vi "test_GUI_with_seq.vi"(8 "Variables":T2=[{"Value"=10.0, "Variable"="dummy", "Save with Image"=FALSE}, {"Value"=-0.0001, "Variable"="HI", "Save with Image"=FALSE}, {"Value"=-0.0002, "Variable"="LO", "Save with Image"=FALSE}, {"Value"=0.0, "Variable"="dummy1", "Save with Image"=FALSE}, {"Value"=0.0, "Variable"="dummy2", "Save with Image"=FALSE}, {"Value"=0.0, "Variable"="dummy3", "Save with Image"=FALSE}, {"Value"=0.0, "Variable"="tLEDuv", "Save with Image"=FALSE}, {"Value"=1000.0, "Variable"="tMOT0", "Save with Image"=FALSE}, {"Value"=20.0, "Variable"="tMOT1", "Save with Image"=FALSE}, {"Value"=40.0, "Variable"="tMOT2", "Save with Image"=FALSE}, {"Value"=50.0, "Variable"="tMOT3", "Save with Image"=FALSE}, {"Value"=13.0, "Variable"="tMOT3delayREP", "Save with Image"=FALSE}, {"Value"=0.05, "Variable"="tREP", "Save with Image"=FALSE}, {"Value"=0.75, "Variable"="dMOT0", "Save with Image"=FALSE}, {"Value"=1.75, "Variable"="dMOT1", "Save with Image"=FALSE}, {"Value"=1.75, "Variable"="dMOT2", "Save with Image"=FALSE}, {"Value"=0.0, "Variable"="dummy5", "Save with Image"=FALSE}, {"Value"=1.45, "Variable"="pMOT0", "Save with Image"=FALSE}, {"Value"=1.45, "Variable"="pMOT1", "Save with Image"=FALSE}, {"Value"=1.25, "Variable"="pMOT2", "Save with Image"=FALSE}, {"Value"=-1.0, "Variable"="dummy6", "Save with Image"=FALSE}, {"Value"=1.6, "Variable"="pRP0", "Save with Image"=FALSE}, {"Value"=1.6, "Variable"="pRP1", "Save with Image"=FALSE}, {"Value"=0.8, "Variable"="pRP2", "Save with Image"=FALSE}, {"Value"=0.0, "Variable"="MOTdummy0", "Save with Image"=FALSE}, {"Value"=-1.0, "Variable"="MOTdummy1", "Save with Image"=FALSE}, {"Value"=0.0, "Variable"="MOTdummy2", "Save with Image"=FALSE}, {"Value"=0.0, "Variable"="MOTdummy3", "Save with Image"=FALSE}, {"Value"=0.0, "Variable"="MOTdummy4", "Save with Image"=FALSE}, {"Value"=1.8, "Variable"="pCROSS0", "Save with Image"=FALSE}, {"Value"=1.29, "Variable"="pCROSS1", "Save with Image"=FALSE}, {"Value"=1.05, "Variable"="pCROSS2", "Save with Image"=FALSE}, {"Value"=0.75, "Variable"="pCROSS3", "Save with Image"=FALSE}, {"Value"=0.0, "Variable"="pCROSS4", "Save with Image"=FALSE}, {"Value"=5.0, "Variable"="pDIMPL0", "Save with Image"=FALSE}, {"Value"=4.4, "Variable"="pDIMPL1", "Save with Image"=FALSE}, {"Value"=3.65, "Variable"="pDIMPL2", "Save with Image"=FALSE}, {"Value"=3.55, "Variable"="pDIMPL3", "Save with Image"=FALSE}, {"Value"=3.45, "Variable"="pDIMPL4", "Save with Image"=FALSE}, {"Value"=1.8, "Variable"="pTightTrap", "Save with Image"=FALSE}, {"Value"=400.0, "Variable"="tHOLD", "Save with Image"=FALSE}, {"Value"=740.0, "Variable"="tEVAP1", "Save with Image"=FALSE}, {"Value"=2900.0, "Variable"="tEVAP2", "Save with Image"=FALSE}, {"Value"=590.0, "Variable"="tEVAP3", "Save with Image"=FALSE}, {"Value"=50.0, "Variable"="tEVAP4", "Save with Image"=FALSE}, {"Value"=50.0, "Variable"="tHOLDTight", "Save with Image"=FALSE}, {"Value"=0.0, "Variable"="ODTdummy1", "Save with Image"=FALSE}, {"Value"=0.0, "Variable"="ODTdummy2", "Save with Image"=FALSE}, {"Value"=0.0, "Variable"="ODTdummy3", "Save with Image"=FALSE}, {"Value"=0.0, "Variable"="ODTdummy4", "Save with Image"=FALSE}, {"Value"=0.0, "Variable"="ODTdummy5", "Save with Image"=FALSE}, {"Value"=3.59, "Variable"="dIMGx", "Save with Image"=FALSE}, {"Value"=3.59, "Variable"="dIMGx0", "Save with Image"=FALSE}, {"Value"=1.38, "Variable"="dIMGz", "Save with Image"=FALSE}, {"Value"=1.98, "Variable"="dEXCz", "Save with Image"=FALSE}, {"Value"=3.0, "Variable"="pABSx", "Save with Image"=FALSE}, {"Value"=1.35, "Variable"="pABSz", "Save with Image"=FALSE}, {"Value"=0.55, "Variable"="pEXCz", "Save with Image"=FALSE}, {"Value"=0.0, "Variable"="TOF", "Save with Image"=FALSE}, {"Value"=10.0, "Variable"="TOFatomFall", "Save with Image"=FALSE}, {"Value"=0.012, "Variable"="tEXP", "Save with Image"=FALSE}, {"Value"=0.2, "Variable"="tEXP2", "Save with Image"=FALSE}, {"Value"=0.082, "Variable"="tEXC", "Save with Image"=FALSE}, {"Value"=0.001, "Variable"="tWaitIoniz", "Save with Image"=FALSE}, {"Value"=0.065, "Variable"="tCAM", "Save with Image"=FALSE}, {"Value"=200.0, "Variable"="tCAMguppy", "Save with Image"=FALSE}, {"Value"=50.0, "Variable"="tCAMreadout", "Save with Image"=FALSE}, {"Value"=-0.002, "Variable"="tTrigDelay", "Save with Image"=FALSE}, {"Value"=0.0, "Variable"="tTrans", "Save with Image"=FALSE}, {"Value"=1.0, "Variable"="tEXCres", "Save with Image"=FALSE}, {"Value"=0.004, "Variable"="tPUMP", "Save with Image"=FALSE}, {"Value"=2.0, "Variable"="pBLUEswitch", "Save with Image"=FALSE}, {"Value"=2.0, "Variable"="pBLUEswitchEIT", "Save with Image"=FALSE}, {"Value"=3.5, "Variable"="dBLUE", "Save with Image"=FALSE}, {"Value"=3.5, "Variable"="dBLUE0", "Save with Image"=FALSE}, {"Value"=1.7, "Variable"="dBLUEdec", "Save with Image"=FALSE}, {"Value"=2.5, "Variable"="dBLUEdec0", "Save with Image"=FALSE}, {"Value"=3.2, "Variable"="dIMPnew", "Save with Image"=FALSE}, {"Value"=1.0, "Variable"="blueON1", "Save with Image"=FALSE}, {"Value"=0.0, "Variable"="blueON2", "Save with Image"=FALSE}, {"Value"=1.0, "Variable"="blueEXCON1", "Save with Image"=FALSE}, {"Value"=0.0, "Variable"="blueEXCON2", "Save with Image"=FALSE}, {"Value"=35.637858, "Variable"="dRydMW", "Save with Image"=FALSE}, {"Value"=16.0, "Variable"="pRydMW", "Save with Image"=FALSE}, {"Value"=50.0, "Variable"="MWduration", "Save with Image"=FALSE}, {"Value"=4.33, "Variable"="bmw0", "Save with Image"=FALSE}, {"Value"=0.02, "Variable"="bmw1", "Save with Image"=FALSE}, {"Value"=0.0, "Variable"="MWdummy1", "Save with Image"=FALSE}, {"Value"=0.0, "Variable"="MWdummy2", "Save with Image"=FALSE}, {"Value"=0.0, "Variable"="MWdummy3", "Save with Image"=FALSE}, {"Value"=4.3, "Variable"="foffset", "Save with Image"=FALSE}, {"Value"=8.64, "Variable"="fdx", "Save with Image"=FALSE}, {"Value"=-5.78, "Variable"="fdy", "Save with Image"=FALSE}, {"Value"=4.0, "Variable"="fdz", "Save with Image"=FALSE}, {"Value"=300.0, "Variable"="CH203", "Save with Image"=FALSE}, {"Value"=160.0, "Variable"="CH215", "Save with Image"=FALSE}, {"Value"=4.0, "Variable"="CH302", "Save with Image"=FALSE}, {"Value"=280.0, "Variable"="CH315", "Save with Image"=FALSE}, {"Value"=0.0, "Variable"="CH202", "Save with Image"=FALSE}, {"Value"=0.0, "Variable"="CH308", "Save with Image"=FALSE}, {"Value"=0.0, "Variable"="EFIELDdummy2", "Save with Image"=FALSE}, {"Value"=0.0, "Variable"="EFIELDdummy3", "Save with Image"=FALSE}, {"Value"=0.0, "Variable"="EFIELDdummy4", "Save with Image"=FALSE}, {"Value"=0.0, "Variable"="EFIELDdummy5", "Save with Image"=FALSE}, {"Value"=0.0, "Variable"="EFIELDdummy6", "Save with Image"=FALSE}, {"Value"=0.0, "Variable"="EFIELDdummy7", "Save with Image"=FALSE}, {"Value"=1.25, "Variable"="bMOT0", "Save with Image"=FALSE}, {"Value"=2.5, "Variable"="bMOT1", "Save with Image"=FALSE}, {"Value"=2.5, "Variable"="bMOT2", "Save with Image"=FALSE}, {"Value"=1.25, "Variable"="bMOT3", "Save with Image"=FALSE}, {"Value"=0.0, "Variable"="bCOMPx", "Save with Image"=FALSE}, {"Value"=1.35, "Variable"="bCOMPy", "Save with Image"=FALSE}, {"Value"=0.27, "Variable"="bCOMPz", "Save with Image"=FALSE}, {"Value"=0.7, "Variable"="bCOMPx1", "Save with Image"=FALSE}, {"Value"=1.1, "Variable"="bCOMPy1", "Save with Image"=FALSE}, {"Value"=0.5, "Variable"="bCOMPz1", "Save with Image"=FALSE}, {"Value"=4.35, "Variable"="bxfinal", "Save with Image"=FALSE}, {"Value"=0.0, "Variable"="byfinal", "Save with Image"=FALSE}, {"Value"=0.0, "Variable"="bzfinal", "Save with Image"=FALSE}, {"Value"=0.0, "Variable"="BFIELDdummy1", "Save with Image"=FALSE}, {"Value"=0.0, "Variable"="BFIELDdummy2", "Save with Image"=FALSE}, {"Value"=0.0, "Variable"="BFIELDdummy3", "Save with Image"=FALSE}, {"Value"=10.0, "Variable"="tCOILsettle", "Save with Image"=FALSE}, {"Value"=0.0, "Variable"="tRemove", "Save with Image"=FALSE}, {"Value"=3.6, "Variable"="pRemove", "Save with Image"=FALSE}, {"Value"=3.1, "Variable"="dF2CLEAN1x", "Save with Image"=FALSE}, {"Value"=20.0, "Variable"="tF2CLEAN1x", "Save with Image"=FALSE}, {"Value"=4.0, "Variable"="tF2CLEAN2x", "Save with Image"=FALSE}, {"Value"=0.0, "Variable"="tDelayDown", "Save with Image"=FALSE}, {"Value"=156.0, "Variable"="oDDSbluePro", "Save with Image"=FALSE}, {"Value"=-10.25, "Variable"="dDDSbluePro", "Save with Image"=FALSE}, {"Value"=50.0, "Variable"="tRampDDSbluePro", "Save with Image"=FALSE}, {"Value"=416.6261, "Variable"="oDDSred", "Save with Image"=FALSE}, {"Value"=-50.25, "Variable"="dDDSred", "Save with Image"=FALSE}, {"Value"=90.0, "Variable"="tRampDDSred", "Save with Image"=FALSE}, {"Value"=154.0, "Variable"="oDDSblueOld", "Save with Image"=FALSE}, {"Value"=10.0, "Variable"="dDDSblueOld", "Save with Image"=FALSE}, {"Value"=100.0, "Variable"="tRampDDSblueOld", "Save with Image"=FALSE}, {"Value"=1.0, "Variable"="mwON", "Save with Image"=FALSE}, {"Value"=9.4e-05, "Variable"="tRabi", "Save with Image"=FALSE}, {"Value"=9.4e-05, "Variable"="tRabi2", "Save with Image"=FALSE}, {"Value"=5e-05, "Variable"="tRamsey", "Save with Image"=FALSE}, {"Value"=0.0, "Variable"="tRamsey2", "Save with Image"=FALSE}, {"Value"=0.0, "Variable"="tDDSa", "Save with Image"=FALSE}, {"Value"=0.0, "Variable"="tDDSb", "Save with Image"=FALSE}, {"Value"=399.942, "Variable"="dDDSa", "Save with Image"=FALSE}, {"Value"=399.942, "Variable"="dDDSa2", "Save with Image"=FALSE}, {"Value"=0.2, "Variable"="pDDSa", "Save with Image"=FALSE}, {"Value"=1e-07, "Variable"="pDDSa2", "Save with Image"=FALSE}, {"Value"=0.0, "Variable"="phiDDSa", "Save with Image"=FALSE}, {"Value"=0.875, "Variable"="phiDDSa2", "Save with Image"=FALSE}, {"Value"=399.942, "Variable"="dDDSb", "Save with Image"=FALSE}, {"Value"=400.009, "Variable"="dDDSb2", "Save with Image"=FALSE}, {"Value"=0.25, "Variable"="pDDSb", "Save with Image"=FALSE}, {"Value"=1e-07, "Variable"="pDDSb2", "Save with Image"=FALSE}, {"Value"=0.25, "Variable"="phiDDSb", "Save with Image"=FALSE}, {"Value"=0.55, "Variable"="phiDDSb2", "Save with Image"=FALSE}, {"Value"=300.0, "Variable"="tDipole", "Save with Image"=FALSE}, {"Value"=0.7, "Variable"="bCOMPx2", "Save with Image"=FALSE}, {"Value"=0.8, "Variable"="bCOMPy2", "Save with Image"=FALSE}, {"Value"=0.6, "Variable"="bCOMPz2", "Save with Image"=FALSE}, {"Value"=20.0, "Variable"="dMOTRamp1", "Save with Image"=FALSE}, {"Value"=18.0, "Variable"="DMOTload", "Save with Image"=FALSE}, {"Value"=50.0, "Variable"="dMOTRamp2", "Save with Image"=FALSE}, {"Value"=272.0, "Variable"="DMOTimag", "Save with Image"=FALSE}, {"Value"=1000.0, "Variable"="oDDShyperfine", "Save with Image"=FALSE}, {"Value"=0.1, "Variable"="dDDShyperfine", "Save with Image"=FALSE}, {"Value"=0.0, "Variable"="tof", "Save with Image"=FALSE}, {"Value"=262.5, "Variable"="dOPump", "Save with Image"=FALSE}, {"Value"=4500.0, "Variable"="tRampOPump", "Save with Image"=FALSE}, {"Value"=10.0, "Variable"="tOPump", "Save with Image"=FALSE}, {"Value"=1.5, "Variable"="bCOMPx3", "Save with Image"=FALSE}, {"Value"=0.8, "Variable"="bCOMPy3", "Save with Image"=FALSE}, {"Value"=0.0, "Variable"="bCOMPz3", "Save with Image"=FALSE}, {"Value"=0.0, "Variable"="bCOMPx4", "Save with Image"=FALSE}, {"Value"=0.0, "Variable"="bCOMPy4", "Save with Image"=FALSE}, {"Value"=0.0, "Variable"="bCOMPz4", "Save with Image"=FALSE}, {"Value"=0.0, "Variable"="scan2photRes", "Save with Image"=FALSE}, {"Value"=0.0, "Variable"="tEXCsmallProbe", "Save with Image"=FALSE}, {"Value"=0.082, "Variable"="tEXCBlue", "Save with Image"=FALSE}, {"Value"=0.0015, "Variable"="tDownPump", "Save with Image"=FALSE}, {"Value"=98.75, "Variable"="RF1freq1", "Save with Image"=FALSE}, {"Value"=0.1, "Variable"="RF1freq2", "Save with Image"=FALSE}, {"Value"=98.75, "Variable"="dummya", "Save with Image"=FALSE}, {"Value"=0.1, "Variable"="dummyb", "Save with Image"=FALSE}, {"Value"=0.5, "Variable"="ttest", "Save with Image"=FALSE}] {"Value" format="%#.9g"}) -> ()   [LabVIEW 2017]
uses:
  sequence_variables.ctl
  Software/Rydberg_Control/TypeDefinition/variables.ctl
  waveform_variables_new.ctl
panel:
  out "x-y":u32=957
  in  "CH2 Phase dif (deg) 2":dbl=90.0
  out "size(s) 4":i32=55008
  out "size(s) 3":i32=55008
  out "error out":errorcluster
  in  "Channel":u16(ring) items=["Channel 1", "Channel 2"]
  out "size(s) 2":i32=3520
  out "output cluster 2":cluster{"String":string, "Value":u16}={"String"="New waveform...", "Value"=5}
  out "output cluster":cluster{"String":string, "Value":u16}={"String"="Readout", "Value"=4}
  out "New waveform index":i32=4
  out "Waveform value array":u16[](array[numeric])=[0, 1, 2, 3, 4]
  out "Waveform name array":string[](array[string])=["Init X", "WAHUHA", "Readout", "Test", "New waveform..."]
  out "Number of Items":u32=4
  out "XY Graph 2":cluster{dbl[], "y":dbl[]}[](graph)
  out "waveform out":T1=[{"Waveform name"="Init X", "sequence duration (us)"=0.0, "Waveform"=[{"Segment number"=0, "frequency"="20", "phase"="0", "amplitude"="", "duration"="", "envelope"=0}, {"Segment number"=0, "frequency"="20", "phase"="0", "amplitude"="", "duration"="", "envelope"=0}]}, {"Waveform name"="WAHUHA", "sequence duration (us)"=0.0, "Waveform"=[{"Segment number"=0, "frequency"="20", "phase"="0", "amplitude"="", "duration"="", "envelope"=0}, {"Segment number"=0, "frequency"="20", "phase"="0", "amplitude"="", "duration"="", "envelope"=0}, {"Segment number"=0, "frequency"="20", "phase"="90", "amplitude"="", "duration"="", "envelope"=0}, {"Segment number"=0, "frequency"="20", "phase"="90", "amplitude"="", "duration"="", "envelope"=0}, {"Segment number"=0, "frequency"="20", "phase"="270", "amplitude"="", "duration"="", "envelope"=0}, {"Segment number"=0, "frequency"="20", "phase"="270", "amplitude"="", "duration"="", "envelope"=0}, {"Segment number"=0, "frequency"="20", "phase"="180", "amplitude"="", "duration"="", "envelope"=0}, {"Segment number"=0, "frequency"="20", "phase"="180", "amplitude"="", "duration"="", "envelope"=0}]}] {"Waveform"."envelope" items=["Square", "Gaussian"]}
  in  "Reference frequency (MHz)":dbl=5.0
  in  "Reference phase (deg)":dbl=90.0
  in  "Save waveform":bool
  in  "Waveform name":u16(ring) items=["Init X", "WAHUHA", "Readout", "New waveform..."]
  in  "Load waveform":bool
  in  "waveform sequence":T1=[{"Waveform name"="InitX", "sequence duration (us)"=0.0, "Waveform"=[{"Segment number"=0, "frequency"="5", "phase"="0", "amplitude"="1", "duration"="ttest", "envelope"=0}]}, {"Waveform name"="WAHUHA", "sequence duration (us)"=0.0, "Waveform"=[{"Segment number"=0, "frequency"="5", "phase"="0", "amplitude"="1", "duration"="1", "envelope"=0}, {"Segment number"=0, "frequency"="5", "phase"="0", "amplitude"="0", "duration"="1", "envelope"=0}, {"Segment number"=0, "frequency"="5", "phase"="90", "amplitude"="1", "duration"="1", "envelope"=0}, {"Segment number"=0, "frequency"="5", "phase"="90", "amplitude"="0", "duration"="1", "envelope"=0}, {"Segment number"=0, "frequency"="5", "phase"="270", "amplitude"="1", "duration"="1", "envelope"=0}, {"Segment number"=0, "frequency"="5", "phase"="270", "amplitude"="0", "duration"="1", "envelope"=0}, {"Segment number"=0, "frequency"="5", "phase"="180", "amplitude"="1", "duration"="1", "envelope"=0}, {"Segment number"=0, "frequency"="5", "phase"="180", "amplitude"="0", "duration"="1", "envelope"=0}]}, {"Waveform name"="Readout", "sequence duration (us)"=0.0, "Waveform"=[{"Segment number"=0, "frequency"="5", "phase"="90", "amplitude"="1", "duration"="1", "envelope"=0}]}] {"Waveform"."envelope" items=["Square", "Gaussian"]}
  out "size(s)":i32=1504
  out "concatenated string 2":string=":FREQ:RAST 5000000000"
  out "Sampling rate":i64=5000000000
  in  "error in":errorcluster
  in  "VISA resource name in":refnum<visa-resource-name>="USB0::0x168C::0x5082::0000217419::INSTR"
  out "appended array":string[](array[string])
  out "output array":u8[](array[numeric])=[0, 8, 51, 8, 103, 8, 154, 8, 205, 8, 1, 9, 52, 9, 102, 9, 153, 9, 203, 9, 253, 9, 47, 10, 96, 10, 145, 10, 193, 10, 242, 10, 33, 11, 80, 11, 127, 11, 173, 11, 218, 11, 7, 12, 51, 12, 94, 12, 137, 12, 179, 12, 220, 12, 5, 13, 45, 13, 83, 13, 121, 13, 158, 13, 194, 13, 230, 13, 8, 14, 41, 14, 74, 14, 105, 14, 135, 14, 164, 14, 192, 14, 219, 14, 245, 14, 14, 15, 38, 15, 60, 15, 81, 15, 102, 15, 121, 15, 138, 15, 155, 15, 170, 15, 184, 15, 197, 15, 208, 15, 219, 15, 228, 15, 235, 15, 242, 15, 247, 15, 251, 15, 254, 15, 255, 15, 255, 15, 254, 15, 251, 15, 247, 15, 242, 15, 235, 15, 228, 15, 219, 15, 208, 15, 197, 15, 184, 15, 170, 15, 155, 15, 138, 15, 121, 15, 102, 15, 81, 15, 60, 15, 38, 15, 14, 15, 245, 14, 219, 14, 192, 14, 164, 14, 135, 14, 105, 14, 74, 14, 41, 14, 8, 14, 230, 13, 194, 13, 158, 13, 121, 13, 83, 13, 45, 13, 5, 13, 220, 12, 179, 12, 137, 12, 94, 12, 51, 12, 7, 12, 218, 11, 173, 11, 127, 11, 80, 11, 33, 11, 242, 10, 193, 10, 145, 10, 96, 10, 47, 10, 253, 9, 203, 9, 153, 9, 102, 9, 52, 9, 1, 9, 205, 8, 154, 8, 103, 8, 51, 8, 0, 8, 205, 7, 153, 7, 102, 7, 51, 7, 255, 6, 204, 6, 154, 6, 103, 6, 53, 6, 3, 6, 209, 5, 160, 5, 111, 5, 63, 5, 14, 5, 223, 4, 176, 4, 129, 4, 83, 4, 38, 4, 249, 3, 205, 3, 162, 3, 119, 3, 77, 3, 36, 3, 251, 2, 211, 2, 173, 2, 135, 2, 98, 2, 62, 2, 26, 2, 248, 1, 215, 1, 182, 1, 151, 1, 121, 1, 92, 1, 64, 1, 37, 1, 11, 1, 242, 0, 218, 0, 196, 0, 175, 0, 154, 0, 135, 0, 118, 0, 101, 0, 86, 0, 72, 0, 59, 0, 48, 0, 37, 0, 28, 0, 21, 0, 14, 0, 9, 0, 5, 0, 2, 0, 1, 0, 1, 0, 2, 0, 5, 0, 9, 0, 14, 0, 21, 0, 28, 0, 37, 0, 48, 0, 59, 0, 72, 0, 86, 0, 101, 0, 118, 0, 135, 0, 154, 0, 175, 0, 196, 0, 218, 0, 242, 0, 11, 1, 37, 1, 64, 1, 92, 1, 121, 1, 151, 1, 182, 1, 215, 1, 248, 1, 26, 2, 62, 2, 98, 2, 135, 2, 173, 2, 211, 2, 251, 2, 36, 3, 77, 3, 119, 3, 162, 3, 205, 3, 249, 3, 38, 4, 83, 4, 129, 4, 176, 4, 223, 4, 14, 5, 63, 5, 111, 5, 160, 5, 209, 5, 3, 6, 53, 6, 103, 6, 154, 6, 204, 6, 255, 6, 51, 7, 102, 7, 153, 7, 205, 7, 0, 8, 51, 8, 103, 8, 154, 8, 205, 8, 1, 9, 52, 9, 102, 9, 153, 9, 203, 9, 253, 9, 47, 10, 96, 10, 145, 10, 193, 10, 242, 10, 33, 11, 80, 11, 127, 11, 173, 11, 218, 11, 7, 12, 51, 12, 94, 12, 137, 12, 179, 12, 220, 12, 5, 13, 45, 13, 83, 13, 121, 13, 158, 13, 194, 13, 230, 13, 8, 14, 41, 14, 74, 14, 105, 14, 135, 14, 164, 14, 192, 14, 219, 14, 245, 14, 14, 15, 38, 15, 60, 15, 81, 15, 102, 15, 121, 15, 138, 15, 155, 15, 170, 15, 184, 15, 197, 15, 208, 15, 219, 15, 228, 15, 235, 15, 242, 15, 247, 15, 251, 15, 254, 15, 255, 15, 255, 15, 254, 15, 251, 15, 247, 15, 242, 15, 235, 15, 228, 15, 219, 15, 208, 15, 197, 15, 184, 15, 170, 15, 155, 15, 138, 15, 121, 15, 102, 15, 81, 15, 60, 15, 38, 15, 14, 15, 245, 14, 219, 14, 192, 14, 164, 14, 135, 14, 105, 14, 74, 14, 41, 14, 8, 14, 230, 13, 194, 13, 158, 13, 121, 13, 83, 13, 45, 13, 5, 13, 220, 12, 179, 12, 137, 12, 94, 12, 51, 12, 7, 12, 218, 11, 173, 11, 127, 11, 80, 11, 33, 11, 242, 10, 193, 10, 145, 10, 96, 10, 47, 10, 253, 9, 203, 9, 153, 9, 102, 9, 52, 9, 1, 9, 205, 8, 154, 8, 103, 8, 51, 8, 0, 8, 205, 7, 153, 7, 102, 7, 51, 7, 255, 6, 204, 6, 154, 6, 103, 6, 53, 6, 3, 6, 209, 5, 160, 5, 111, 5, 63, 5, 14, 5, 223, 4, 176, 4, 129, 4, 83, 4, 38, 4, 249, 3, 205, 3, 162, 3, 119, 3, 77, 3, 36, 3, 251, 2, 211, 2, 173, 2, 135, 2, 98, 2, 62, 2, 26, 2, 248, 1, 215, 1, 182, 1, 151, 1, 121, 1, 92, 1, 64, 1, 37, 1, 11, 1, 242, 0, 218, 0, 196, 0, 175, 0, 154, 0, 135, 0, 118, 0, 101, 0, 86, 0, 72, 0, 59, 0, 48, 0, 37, 0, 28, 0, 21, 0, 14, 0, 9, 0, 5, 0, 2, 0, 1, 0, 1, 0, 2, 0, 5, 0, 9, 0, 14, 0, 21, 0, 28, 0, 37, 0, 48, 0, 59, 0, 72, 0, 86, 0, 101, 0, 118, 0, 135, 0, 154, 0, 175, 0, 196, 0, 218, 0, 242, 0, 11, 1, 37, 1, 64, 1, 92, 1, 121, 1, 151, 1, 182, 1, 215, 1, 248, 1, 26, 2, 62, 2, 98, 2, 135, 2, 173, 2, 211, 2, 251, 2, 36, 3, 77, 3, 119, 3, 162, 3, 205, 3, 249, 3, 38, 4, 83, 4, 129, 4, 176, 4, 223, 4, 14, 5, 63, 5, 111, 5, 160, 5, 209, 5, 3, 6, 53, 6, 103, 6, 154, 6, 204, 6, 255, 6, 51, 7, 102, 7, 153, 7, 205, 7, 0, 8, 51, 8, 103, 8, 154, 8, 205, 8, 1, 9, 52, 9, 102, 9, 153, 9, 203, 9, 253, 9, 47, 10, 96, 10, 145, 10, 193, 10, 242, 10, 33, 11, 80, 11, 127, 11, 173, 11, 218, 11, 7, 12, 51, 12, 94, 12, 137, 12, 179, 12, 220, 12, 5, 13, 45, 13, 83, 13, 121, 13, 158, 13, 194, 13, 230, 13, 8, 14, 41, 14, 74, 14, 105, 14, 135, 14, 164, 14, 192, 14, 219, 14, 245, 14, 14, 15, 38, 15, 60, 15, 81, 15, 102, 15, 121, 15, 138, 15, 155, 15, 170, 15, 184, 15, 197, 15, 208, 15, 219, 15, 228, 15, 235, 15, 242, 15, 247, 15, 251, 15, 254, 15, 255, 15, 255, 15, 254, 15, 251, 15, 247, 15, 242, 15, 235, 15, 228, 15, 219, 15, 208, 15, 197, 15, 184, 15, 170, 15, 155, 15, 138, 15, 121, 15, 102, 15, 81, 15, 60, 15, 38, 15, 14, 15, 245, 14, 219, 14, 192, 14, 164, 14, 135, 14, 105, 14, 74, 14, 41, 14, 8, 14, 230, 13, 194, 13, 158, 13, 121, 13, 83, 13, 45, 13, 5, 13, 220, 12, 179, 12, 137, 12, 94, 12, 51, 12, 7, 12, 218, 11, 173, 11, 127, 11, 80, 11, 33, 11, 242, 10, 193, 10, 145, 10, 96, 10, 47, 10, 253, 9, 203, 9, 153, 9, 102, 9, 52, 9, 1, 9, 205, 8, 154, 8, 103, 8, 51, 8, 0, 8, 205, 7, 153, 7, 102, 7, 51, 7, 255, 6, 204, 6, 154, 6, 103, 6, 53, 6, 3, 6, 209, 5, 160, 5, 111, 5, 63, 5, 14, 5, 223, 4, 176, 4, 129, 4, 83, 4, 38, 4, 249, 3, 205, 3, 162, 3, 119, 3, 77, 3, 36, 3, 251, 2, 211, 2, 173, 2, 135, 2, 98, 2, 62, 2, 26, 2, 248, 1, 215, 1, 182, 1, 151, 1, 121, 1, 92, 1, 64, 1, 37, 1, 11, 1, 242, 0, 218, 0, 196, 0, 175, 0, 154, 0, 135, 0, 118, 0, 101, 0, 86, 0, 72, 0, 59, 0, 48, 0, 37, 0, 28, 0, 21, 0, 14, 0, 9, 0, 5, 0, 2, 0, 1, 0, 1, 0, 2, 0, 5, 0, 9, 0, 14, 0, 21, 0, 28, 0, 37, 0, 48, 0, 59, 0, 72, 0, 86, 0, 101, 0, 118, 0, 135, 0, 154, 0, 175, 0, 196, 0, 218, 0, 242, 0, 11, 1, 37, 1, 64, 1, 92, 1, 121, 1, 151, 1, 182, 1, 215, 1, 248, 1, 26, 2, 62, 2, 98, 2, 135, 2, 173, 2, 211, 2, 251, 2, 36, 3, 77, 3, 119, 3, 162, 3, 205, 3, 249, 3, 38, 4, 83, 4, 129, 4, 176, 4, 223, 4, 14, 5, 63, 5, 111, 5, 160, 5, 209, 5, 3, 6, 53, 6, 103, 6, 154, 6, 204, 6, 255, 6, 51, 7, 102, 7, 153, 7, 205, 7, 0, 8, 51, 8, 103, 8, 154, 8, 205, 8, 1, 9, 52, 9, 102, 9, 153, 9, 203, 9, 253, 9, 47, 10, 96, 10, 145, 10, 193, 10, 242, 10, 33, 11, 80, 11, 127, 11, 173, 11, 218, 11, 7, 12, 51, 12, 94, 12, 137, 12, 179, 12, 220, 12, 5, 13, 45, 13, 83, 13, 121, 13, 158, 13, 194, 13, 230, 13, 8, 14, 41, 14, 74, 14, 105, 14, 135, 14, 164, 14, 192, 14, 219, 14, 245, 14, 14, 15, 38, 15, 60, 15, 81, 15, 102, 15, 121, 15, 138, 15, 155, 15, 170, 15, 184, 15, 197, 15, 208, 15, 219, 15, 228, 15, 235, 15, 242, 15, 247, 15, 251, 15, 254, 15, 255, 15, 255, 15, 254, 15, 251, 15, 247, 15, 242, 15, 235, 15, 228, 15, 219, 15, 208, 15, 197, 15, 184, 15, 170, 15, 155, 15, 138, 15, 121, 15, 102, 15, 81, 15, 60, 15, 38, 15, 14, 15, 245, 14, 219, 14, 192, 14, 164, 14, 135, 14, 105, 14, 74, 14, 41, 14, 8, 14, 230, 13, 194, 13, 158, 13, 121, 13, 83, 13, 45, 13, 5, 13, 220, 12, 179, 12, 137, 12, 94, 12, 51, 12, 7, 12, 218, 11, 173, 11, 127, 11, 80, 11, 33, 11, 242, 10, 193, 10, 145, 10, 96, 10, 47, 10, 253, 9, 203, 9, 153, 9, 102, 9, 52, 9, 1, 9, 205, 8, 154, 8, 103, 8, 51, 8, 0, 8, 205, 7, 153, 7, 102, 7, 51, 7, 255, 6, 204, 6, 154, 6, 103, 6, 53, 6, 3, 6, 209, 5, 160, 5, 111, 5, 63, 5, 14, 5, 223, 4, 176, 4, 129, 4, 83, 4, 38, 4, 249, 3, 205, 3, 162, 3, 119, 3, 77, 3, 36, 3, 251, 2, 211, 2, 173, 2, 135, 2, 98, 2, 62, 2, 26, 2, 248, 1, 215, 1, 182, 1, 151, 1, 121, 1, 92, 1, 64, 1, 37, 1, 11, 1, 242, 0, 218, 0, 196, 0, 175, 0, 154, 0, 135, 0, 118, 0, 101, 0, 86, 0, 72, 0, 59, 0, 48, 0, 37, 0, 28, 0, 21, 0, 14, 0, 9, 0, 5, 0, 2, 0, 1, 0, 1, 0, 2, 0, 5, 0, 9, 0, 14, 0, 21, 0, 28, 0, 37, 0, 48, 0, 59, 0, 72, 0, 86, 0, 101, 0, 118, 0, 135, 0, 154, 0, 175, 0, 196, 0, 218, 0, 242, 0, 11, 1, 37, 1, 64, 1, 92, 1, 121, 1, 151, 1, 182, 1, 215, 1, 248, 1, 26, 2, 62, 2, 98, 2, 135, 2, 173, 2, 211, 2, 251, 2, 36, 3, 77, 3, 119, 3, 162, 3, 205, 3, 249, 3, 38, 4, 83, 4, 129, 4, 176, 4, 223, 4, 14, 5, 63, 5, 111, 5, 160, 5, 209, 5, 3, 6, 53, 6, 103, 6, 154, 6, 204, 6, 255, 6, 51, 7, 102, 7, 153, 7, 205, 7, 0, 8, 51, 8, 103, 8, 154, 8, 205, 8, 1, 9, 52, 9, 102, 9, 153, 9, 203, 9, 253, 9, 47, 10, 96, 10, 145, 10, 193, 10, 242, 10, 33, 11, 80, 11, 127, 11, 173, 11, 218, 11, 7, 12, 51, 12, 94, 12, 137, 12, 179, 12, 220, 12, 5, 13, 45, 13, 83, 13, 121, 13, 158, 13, 194, 13, 230, 13, 8, 14, 41, 14, 74, 14, 105, 14, 135, 14, 164, 14, 192, 14, 219, 14, 245, 14, 14, 15, 38, 15, 60, 15, 81, 15, 102, 15, 121, 15, 138, 15, 155, 15, 170, 15, 184, 15, 197, 15, 208, 15, 219, 15, 228, 15, 235, 15, 242, 15, 247, 15, 251, 15, 254, 15, 255, 15, 255, 15, 254, 15, 251, 15, 247, 15, 242, 15, 235, 15, 228, 15, 219, 15, 208, 15, 197, 15, 184, 15, 170, 15, 155, 15, 138, 15, 121, 15, 102, 15, 81, 15, 60, 15, 38, 15, 14, 15, 245, 14, 219, 14, 192, 14, 164, 14, 135, 14, 105, 14, 74, 14, 41, 14, 8, 14, 230, 13, 194, 13, 158, 13, 121, 13, 83, 13, 45, 13, 5, 13, 220, 12, 179, 12, 137, 12, 94, 12, 51, 12, 7, 12, 218, 11, 173, 11, 127, 11, 80, 11, 33, 11, 242, 10, 193, 10, 145, 10, 96, 10, 47, 10, 253, 9, 203, 9, 153, 9, 102, 9, 52, 9, 1, 9, 205, 8, 154, 8, 103, 8, 51, 8, 0, 8, 205, 7, 153, 7, 102, 7, 51, 7, 255, 6, 204, 6, 154, 6, 103, 6, 53, 6, 3, 6, 209, 5, 160, 5, 111, 5, 63, 5, 14, 5, 223, 4, 176, 4, 129, 4, 83, 4, 38, 4, 249, 3, 205, 3, 162, 3, 119, 3, 77, 3, 36, 3, 251, 2, 211, 2, 173, 2, 135, 2, 98, 2, 62, 2, 26, 2, 248, 1, 215, 1, 182, 1, 151, 1, 121, 1, 92, 1, 64, 1, 37, 1, 11, 1, 242, 0, 218, 0, 196, 0, 175, 0, 154, 0, 135, 0, 118, 0, 101, 0, 86, 0, 72, 0, 59, 0, 48, 0, 37, 0, 28, 0, 21, 0, 14, 0, 9, 0, 5, 0, 2, 0, 1, 0, 1, 0, 2, 0, 5, 0, 9, 0, 14, 0, 21, 0, 28, 0, 37, 0, 48, 0, 59, 0, 72, 0, 86, 0, 101, 0, 118, 0, 135, 0, 154, 0, 175, 0, 196, 0, 218, 0, 242, 0, 11, 1, 37, 1, 64, 1, 92, 1, 121, 1, 151, 1, 182, 1, 215, 1, 248, 1, 26, 2, 62, 2, 98, 2, 135, 2, 173, 2, 211, 2, 251, 2, 36, 3, 77, 3, 119, 3, 162, 3, 205, 3, 249, 3, 38, 4, 83, 4, 129, 4, 176, 4, 223, 4, 14, 5, 63, 5, 111, 5, 160, 5, 209, 5, 3, 6, 53, 6, 103, 6, 154, 6, 204, 6, 255, 6, 51, 7, 102, 7, 153, 7, 205, 7, 0, 8, 51, 8, 103, 8, 154, 8, 205, 8, 1, 9, 52, 9, 102, 9, 153, 9, 203, 9, 253, 9, 47, 10, 96, 10, 145, 10, 193, 10, 242, 10, 33, 11, 80, 11, 127, 11, 173, 11, 218, 11, 7, 12, 51, 12, 94, 12, 137, 12, 179, 12, 220, 12, 5, 13, 45, 13, 83, 13, 121, 13, 158, 13, 194, 13, 230, 13, 8, 14, 41, 14, 74, 14, 105, 14, 135, 14, 164, 14, 192, 14, 219, 14, 245, 14, 14, 15, 38, 15, 60, 15, 81, 15, 102, 15, 121, 15, 138, 15, 155, 15, 170, 15, 184, 15, 197, 15, 208, 15, 219, 15, 228, 15, 235, 15, 242, 15, 247, 15, 251, 15, 254, 15, 255, 15, 255, 15, 254, 15, 251, 15, 247, 15, 242, 15, 235, 15, 228, 15, 219, 15, 208, 15, 197, 15, 184, 15, 170, 15, 155, 15, 138, 15, 121, 15, 102, 15, 81, 15, 60, 15, 38, 15, 14, 15, 245, 14, 219, 14, 192, 14, 164, 14, 135, 14, 105, 14, 74, 14, 41, 14, 8, 14, 230, 13, 194, 13, 158, 13, 121, 13, 83, 13, 45, 13, 5, 13, 220, 12, 179, 12, 137, 12, 94, 12, 51, 12, 7, 12, 218, 11, 173, 11, 127, 11, 80, 11, 33, 11, 242, 10, 193, 10, 145, 10, 96, 10, 47, 10, 253, 9, 203, 9, 153, 9, 102, 9, 52, 9, 1, 9, 205, 8, 154, 8, 103, 8, 51, 8, 0, 8, 205, 7, 153, 7, 102, 7, 51, 7, 255, 6, 204, 6, 154, 6, 103, 6, 53, 6, 3, 6, 209, 5, 160, 5, 111, 5, 63, 5, 14, 5, 223, 4, 176, 4, 129, 4, 83, 4, 38, 4, 249, 3, 205, 3, 162, 3, 119, 3, 77, 3, 36, 3, 251, 2, 211, 2, 173, 2, 135, 2, 98, 2, 62, 2, 26, 2, 248, 1, 215, 1, 182, 1, 151, 1, 121, 1, 92, 1, 64, 1, 37, 1, 11, 1, 242, 0, 218, 0, 196, 0, 175, 0, 154, 0, 135, 0, 118, 0, 101, 0, 86, 0, 72, 0, 59, 0, 48, 0, 37, 0, 28, 0, 21, 0, 14, 0, 9, 0, 5, 0, 2, 0, 1, 0, 1, 0, 2, 0, 5, 0, 9, 0, 14, 0, 21, 0, 28, 0, 37, 0, 48, 0, 59, 0, 72, 0, 86, 0, 101, 0, 118, 0, 135, 0, 154, 0, 175, 0, 196, 0, 218, 0, 242, 0, 11, 1, 37, 1, 64, 1, 92, 1, 121, 1, 151, 1, 182, 1, 215, 1, 248, 1, 26, 2, 62, 2, 98, 2, 135, 2, 173, 2, 211, 2, 251, 2, 36, 3, 77, 3, 119, 3, 162, 3, 205, 3, 249, 3, 38, 4, 83, 4, 129, 4, 176, 4, 223, 4, 14, 5, 63, 5, 111, 5, 160, 5, 209, 5, 3, 6, 53, 6, 103, 6, 154, 6, 204, 6, 255, 6, 51, 7, 102, 7, 153, 7, 205, 7, 0, 8, 0, 8, 0, 8, 0, 8]
  out "concatenated string":string="*OPC?;:TRAC:DATA#43008"
  out "waveform":dbl[](array[numeric])=[0.0, 0.7246531301870466, 0.7417417727387392, 0.7583619152887219, 0.7745030601987338, 0.7901550123756903, 0.8053078857111219, 0.8199521093254523, 0.8340784336131711, 0.8476779360850831, 0.8607420270039435, 0.8732624548099202, 0.8852313113324551, 0.8966410367852359, 0.9074844245411169, 0.9177546256839811, 0.9274451533346614, 0.9365498867481924, 0.9450630751798048, 0.9529793415172189, 0.9602936856769431, 0.967001487762435, 0.9730985109821265, 0.9785809043254721, 0.9834452049953297, 0.9876883405951378, 0.9913076310695066, 0.9943007903969989, 0.9966659280340299, 0.998401550108975, 0.9995065603657316, 0.9999802608561371, 0.999822352380809, 0.9990329346781247, 0.9976125063612252, 0.99556196460308, 0.9928826045698137, 0.989576118602651, 0.985644595148998, 0.9810905174433341, 0.9759167619387474, 0.9701265964901058, 0.9637236782900097, 0.9567120515588304, 0.9490961449902946, 0.9408807689542255, 0.932071112458211, 0.9226727398701149, 0.9126915874035029, 0.902133959368203, 0.8910065241883679, 0.8793163101905562, 0.8670707011644899, 0.8542774316992952, 0.8409445822981692, 0.8270805742745617, 0.8126941644330941, 0.797794439538571, 0.7823908105765882, 0.7664930068093498, 0.7501110696304594, 0.7332553462225603, 0.7159364830218313, 0.6981654189934726, 0.679953378722419, 0.6613118653236518, 0.6422526531765845, 0.6227877804881126, 0.6029295416890246, 0.5826904796685761, 0.5620833778521305, 0.5411212521268759, 0.5198173426207093, 0.4981851053394905, 0.4762382036679394, 0.45399049973954686, 0.43145604568095886, 0.40864907473634915, 0.3855839922773965, 0.3622753667045458, 0.3387379202452913, 0.31498651965530494, 0.29103616682827177, 0.26690198932037573, 0.2425992307954074, 0.21814324139654231, 0.19354946805086026, 0.16883344471273365, 0.14401078255225216, 0.11909716009486954, 0.09410831331851435, 0.06906002571440606, 0.04396811831786495, 0.01884843971540846, -0.006283143965558882, -0.03141075907812844, -0.056518534482024436, -0.08159061156815768, -0.1066111542752598, -0.13156435909228262, -0.15643446504023073, -0.18120576362713745, -0.2058626087698812, -0.23038942667659065, -0.25477072568338244, -0.2789911060392293, -0.3030352696327742, -0.3268880296549425, -0.35053432019125924, -0.37395920573780045, -0.3971478906347804, -0.42008572841180625, -0.44275823103890133, -0.4651510780774583, -0.48725012572533244, -0.5090414157503717, -0.5305111843067342, -0.5516458706284302, -0.572432125594591, -0.5928568201610591, -0.6129070536529766, -0.6325701619131244, -0.6518337253008785, -0.6706855765367199, -0.6891138083873485, -0.7071067811865477, -0.7246531301870467, -0.7417417727387394, -0.7583619152887215, -0.7745030601987337, -0.7901550123756904, -0.8053078857111221, -0.8199521093254526, -0.834078433613171, -0.8476779360850837, -0.8607420270039438, -0.8732624548099199, -0.8852313113324551, -0.8966410367852359, -0.907484424541117, -0.9177546256839813, -0.9274451533346612, -0.9365498867481923, -0.9450630751798049, -0.9529793415172186, -0.960293685676943, -0.967001487762435, -0.9730985109821266, -0.9785809043254722, -0.9834452049953297, -0.9876883405951379, -0.9913076310695065, -0.9943007903969988, -0.9966659280340299, -0.998401550108975, -0.9995065603657316, -0.9999802608561371, -0.999822352380809, -0.9990329346781247, -0.9976125063612252, -0.99556196460308, -0.9928826045698137, -0.989576118602651, -0.985644595148998, -0.9810905174433341, -0.9759167619387475, -0.9701265964901059, -0.9637236782900097, -0.9567120515588304, -0.9490961449902945, -0.9408807689542253, -0.9320711124582107, -0.9226727398701148, -0.9126915874035028, -0.9021339593682026, -0.891006524188368, -0.8793163101905562, -0.8670707011644899, -0.8542774316992949, -0.8409445822981693, -0.8270805742745618, -0.8126941644330938, -0.7977944395385713, -0.7823908105765883, -0.7664930068093498, -0.7501110696304595, -0.7332553462225604, -0.7159364830218313, -0.6981654189934727, -0.6799533787224191, -0.6613118653236516, -0.642252653176584, -0.6227877804881126, -0.6029295416890247, -0.5826904796685758, -0.5620833778521301, -0.541121252126876, -0.5198173426207094, -0.4981851053394906, -0.4762382036679395, -0.45399049973954697, -0.43145604568095897, -0.40864907473634887, -0.385583992277397, -0.3622753667045459, -0.3387379202452914, -0.31498651965530466, -0.2910361668282715, -0.266901989320375, -0.24259923079540666, -0.21814324139654243, -0.19354946805085993, -0.16883344471273334, -0.1440107825522523, -0.11909716009486966, -0.09410831331851403, -0.0690600257144053, -0.043968118317865075, -0.018848439715408137, 0.0062831439655592035, 0.03141075907812787, 0.05651853448202431, 0.08159061156815756, 0.10661115427526012, 0.13156435909228203, 0.15643446504023062, 0.1812057636271373, 0.2058626087698815, 0.23038942667659096, 0.25477072568338277, 0.27899110603923005, 0.3030352696327741, 0.3268880296549428, 0.3505343201912595, 0.37395920573780034, 0.3971478906347807, 0.4200857284118065, 0.4427582310389012, 0.4651510780774582, 0.4872501257253324, 0.5090414157503715, 0.5305111843067337, 0.5516458706284301, 0.5724321255945909, 0.5928568201610587, 0.6129070536529762, 0.6325701619131243, 0.6518337253008788, 0.6706855765367201, 0.6891138083873487, 0.7071067811865479, 0.7246531301870466, 0.7417417727387393, 0.7583619152887221, 0.7745030601987342, 0.7901550123756903, 0.805307885711122, 0.8199521093254525, 0.834078433613171, 0.8476779360850831, 0.8607420270039436, 0.8732624548099203, 0.885231311332455, 0.8966410367852358, 0.907484424541117, 0.9177546256839809, 0.9274451533346612, 0.9365498867481926, 0.9450630751798051, 0.9529793415172189, 0.9602936856769432, 0.9670014877624352, 0.9730985109821265, 0.9785809043254722, 0.9834452049953296, 0.9876883405951377, 0.9913076310695066, 0.9943007903969989, 0.9966659280340299, 0.998401550108975, 0.9995065603657316, 0.9999802608561371, 0.9998223523808091, 0.9990329346781247, 0.9976125063612252, 0.99556196460308, 0.9928826045698136, 0.9895761186026509, 0.985644595148998, 0.9810905174433341, 0.9759167619387473, 0.9701265964901057, 0.9637236782900095, 0.9567120515588302, 0.9490961449902943, 0.9408807689542257, 0.9320711124582111, 0.9226727398701149, 0.9126915874035028, 0.9021339593682027, 0.8910065241883676, 0.8793163101905568, 0.8670707011644905, 0.8542774316992955, 0.8409445822981693, 0.8270805742745619, 0.812694164433094, 0.7977944395385709, 0.7823908105765889, 0.7664930068093494, 0.7501110696304601, 0.7332553462225593, 0.7159364830218314, 0.6981654189934715, 0.6799533787224192, 0.661311865323653, 0.6422526531765841, 0.6227877804881135, 0.602929541689024, 0.5826904796685767, 0.5620833778521296, 0.5411212521268761, 0.5198173426207111, 0.49818510533949073, 0.4762382036679404, 0.4539904997395463, 0.4314560456809599, 0.40864907473634815, 0.3855839922773971, 0.3622753667045477, 0.33873792024529153, 0.31498651965530644, 0.2910361668282716, 0.26690198932037684, 0.24259923079540677, 0.21814324139654342, 0.19354946805085918, 0.16883344471273434, 0.14401078255225067, 0.11909716009486979, 0.09410831331851238, 0.06906002571440542, 0.043968118317862535, 0.01884843971540737, -0.006283143965558193, -0.03141075907812952, -0.056518534482024194, -0.08159061156815921, -0.10661115427526001, -0.13156435909228456, -0.15643446504023137, -0.18120576362713633, -0.20586260876988224, -0.23038942667659, -0.2547707256833835, -0.27899110603922905, -0.30303526963277566, -0.3268880296549427, -0.35053432019125774, -0.37395920573780106, -0.3971478906347798, -0.42008572841180725, -0.4427582310389011, -0.4651510780774597, -0.4872501257253323, -0.5090414157503699, -0.5305111843067344, -0.5516458706284292, -0.5724321255945916, -0.5928568201610586, -0.6129070536529775, -0.6325701619131242, -0.6518337253008772, -0.6706855765367201, -0.6891138083873474, -0.7071067811865479, -0.7246531301870459, -0.7417417727387399, -0.7583619152887214, -0.7745030601987347, -0.7901550123756902, -0.805307885711123, -0.8199521093254525, -0.8340784336131724, -0.8476779360850836, -0.8607420270039432, -0.8732624548099207, -0.8852313113324549, -0.8966410367852365, -0.9074844245411169, -0.9177546256839819, -0.9274451533346615, -0.936549886748192, -0.945063075179805, -0.9529793415172185, -0.9602936856769434, -0.967001487762435, -0.973098510982127, -0.9785809043254721, -0.9834452049953294, -0.9876883405951378, -0.9913076310695064, -0.994300790396999, -0.9966659280340299, -0.9984015501089751, -0.9995065603657316, -0.9999802608561371, -0.999822352380809, -0.9990329346781248, -0.9976125063612251, -0.9955619646030801, -0.9928826045698136, -0.989576118602651, -0.9856445951489978, -0.9810905174433341, -0.975916761938747, -0.9701265964901058, -0.963723678290009, -0.9567120515588303, -0.9490961449902948, -0.9408807689542251, -0.9320711124582112, -0.9226727398701142, -0.9126915874035028, -0.902133959368202, -0.8910065241883677, -0.8793163101905568, -0.8670707011644896, -0.8542774316992955, -0.8409445822981684, -0.8270805742745619, -0.812694164433093, -0.7977944395385709, -0.782390810576589, -0.7664930068093495, -0.7501110696304601, -0.7332553462225594, -0.7159364830218315, -0.6981654189934716, -0.6799533787224193, -0.6613118653236532, -0.6422526531765842, -0.6227877804881135, -0.6029295416890241, -0.5826904796685768, -0.5620833778521297, -0.5411212521268762, -0.5198173426207112, -0.49818510533949084, -0.4762382036679405, -0.4539904997395464, -0.43145604568096, -0.40864907473634826, -0.3855839922773972, -0.3622753667045445, -0.33873792024529165, -0.3149865196553032, -0.2910361668282717, -0.2669019893203735, -0.2425992307954069, -0.21814324139654007, -0.19354946805085932, -0.16883344471273445, -0.14401078255225078, -0.1190971600948699, -0.09410831331851251, -0.06906002571440555, -0.04396811831786266, -0.018848439715407492, 0.006283143965558071, 0.0314107590781294, 0.05651853448202407, 0.08159061156815908, 0.10661115427525988, 0.13156435909228092, 0.15643446504023126, 0.1812057636271362, 0.20586260876988213, 0.23038942667658985, 0.2547707256833834, 0.27899110603922894, 0.30303526963277216, 0.32688802965494257, 0.35053432019125763, 0.37395920573780095, 0.3971478906347797, 0.42008572841180714, 0.442758231038901, 0.4651510780774564, 0.48725012572533216, 0.5090414157503698, 0.5305111843067343, 0.5516458706284291, 0.5724321255945914, 0.5928568201610586, 0.6129070536529774, 0.6325701619131241, 0.6518337253008799, 0.67068557653672, 0.6891138083873498, 0.7071067811865478, 0.7246531301870482, 0.7417417727387398, 0.7583619152887213, 0.7745030601987346, 0.7901550123756902, 0.8053078857111229, 0.8199521093254524, 0.8340784336131724, 0.8476779360850835, 0.8607420270039431, 0.8732624548099206, 0.8852313113324549, 0.8966410367852364, 0.9074844245411169, 0.9177546256839818, 0.9274451533346614, 0.9365498867481918, 0.945063075179805, 0.9529793415172185, 0.9602936856769434, 0.9670014877624349, 0.9730985109821269, 0.9785809043254721, 0.9834452049953294, 0.9876883405951378, 0.9913076310695064, 0.9943007903969989, 0.9966659280340299, 0.9984015501089751, 0.9995065603657316, 0.9999802608561371, 0.999822352380809, 0.9990329346781248, 0.9976125063612252, 0.9955619646030798, 0.9928826045698136, 0.989576118602651, 0.9856445951489978, 0.9810905174433341, 0.975916761938747, 0.9701265964901058, 0.9637236782900092, 0.9567120515588303, 0.9490961449902949, 0.9408807689542251, 0.9320711124582112, 0.9226727398701142, 0.9126915874035029, 0.9021339593682021, 0.8910065241883677, 0.8793163101905551, 0.8670707011644897, 0.8542774316992937, 0.8409445822981685, 0.827080574274562, 0.8126941644330931, 0.797794439538571, 0.7823908105765869, 0.7664930068093495, 0.7501110696304579, 0.7332553462225594, 0.7159364830218317, 0.6981654189934717, 0.6799533787224193, 0.6613118653236506, 0.6422526531765842, 0.6227877804881108, 0.6029295416890242, 0.5826904796685769, 0.5620833778521298, 0.5411212521268763, 0.5198173426207082, 0.49818510533949095, 0.47623820366793745, 0.4539904997395465, 0.43145604568096013, 0.40864907473634837, 0.3855839922773973, 0.36227536670454463, 0.33873792024529176, 0.31498651965530333, 0.2910361668282718, 0.26690198932037706, 0.24259923079540702, 0.21814324139654367, 0.19354946805085943, 0.16883344471273456, 0.1440107825522509, 0.11909716009487002, 0.09410831331851616, 0.06906002571440566, 0.04396811831786633, 0.018848439715407617, -0.0062831439655579475, -0.03141075907812928, -0.05651853448202395, -0.08159061156815542, -0.10661115427525976, -0.13156435909228079, -0.15643446504023115, -0.18120576362713608, -0.20586260876987852, -0.23038942667658974, -0.25477072568337983, -0.27899110603922883, -0.30303526963277205, -0.32688802965494246, -0.3505343201912575, -0.37395920573780084, -0.39714789063477957, -0.420085728411807, -0.4427582310389009, -0.4651510780774595, -0.48725012572533205, -0.5090414157503728, -0.5305111843067342, -0.551645870628432, -0.5724321255945913, -0.5928568201610612, -0.6129070536529773, -0.6325701619131268, -0.6518337253008798, -0.6706855765367199, -0.6891138083873498, -0.7071067811865477, -0.7246531301870481, -0.7417417727387396, -0.7583619152887235, -0.7745030601987345, -0.7901550123756901, -0.8053078857111229, -0.8199521093254523, -0.8340784336131722, -0.8476779360850835, -0.8607420270039449, -0.8732624548099206, -0.8852313113324549, -0.8966410367852364, -0.9074844245411168, -0.9177546256839818, -0.9274451533346614, -0.9365498867481931, -0.945063075179805, -0.9529793415172185, -0.9602936856769433, -0.9670014877624349, -0.9730985109821269, -0.9785809043254721, -0.9834452049953301, -0.9876883405951378, -0.9913076310695064, -0.9943007903969989, -0.9966659280340298, -0.9984015501089751, -0.9995065603657315, -0.9999802608561371, -0.999822352380809, -0.9990329346781248, -0.9976125063612252, -0.9955619646030801, -0.9928826045698136, -0.989576118602651, -0.9856445951489978, -0.9810905174433342, -0.9759167619387478, -0.9701265964901058, -0.9637236782900102, -0.9567120515588303, -0.9490961449902949, -0.9408807689542251, -0.93207111245821, -0.9226727398701143, -0.9126915874035014, -0.9021339593682021, -0.8910065241883661, -0.8793163101905552, -0.867070701164488, -0.8542774316992938, -0.8409445822981685, -0.8270805742745602, -0.8126941644330931, -0.7977944395385689, -0.782390810576587, -0.7664930068093474, -0.750111069630458, -0.7332553462225595, -0.7159364830218292, -0.6981654189934718, -0.6799533787224169, -0.6613118653236507, -0.6422526531765816, -0.6227877804881109, -0.6029295416890244, -0.5826904796685741, -0.5620833778521299, -0.5411212521268735, -0.5198173426207083, -0.49818510533948795, -0.47623820366793757, -0.45399049973954664, -0.431456045680957, -0.4086490747363485, -0.38558399227739415, -0.36227536670454474, -0.33873792024528854, -0.31498651965530344, -0.29103616682827194, -0.2669019893203738, -0.24259923079540713, -0.21814324139654032, -0.19354946805085954, -0.1688334447127312, -0.14401078255225103, -0.11909716009487015, -0.09410831331851274, -0.06906002571440578, -0.0439681183178629, -0.018848439715407738, 0.006283143965561378, 0.03141075907812916, 0.056518534482023826, 0.08159061156815883, 0.10661115427525963, 0.1315643590922842, 0.156434465040231, 0.18120576362713944, 0.20586260876988188, 0.23038942667658963, 0.25477072568338316, 0.2789911060392287, 0.30303526963277533, 0.32688802965494235, 0.35053432019126074, 0.37395920573780067, 0.39714789063477945, 0.4200857284118069, 0.4427582310389008, 0.46515107807745937, 0.48725012572533194, 0.5090414157503726, 0.530511184306734, 0.551645870628429, 0.5724321255945912, 0.5928568201610583, 0.6129070536529772, 0.6325701619131239, 0.6518337253008797, 0.6706855765367198, 0.6891138083873497, 0.7071067811865476, 0.7246531301870481, 0.7417417727387395, 0.7583619152887235, 0.7745030601987344, 0.7901550123756922, 0.8053078857111228, 0.8199521093254543, 0.8340784336131722, 0.8476779360850852, 0.8607420270039448, 0.8732624548099223, 0.8852313113324565, 0.8966410367852363, 0.9074844245411182, 0.9177546256839818, 0.9274451533346626, 0.9365498867481931, 0.9450630751798049, 0.9529793415172195, 0.9602936856769433, 0.9670014877624358, 0.9730985109821269, 0.9785809043254727, 0.98344520499533, 0.9876883405951378, 0.9913076310695068, 0.9943007903969989, 0.9966659280340301, 0.9984015501089751, 0.9995065603657316, 0.9999802608561371, 0.999822352380809, 0.9990329346781246, 0.9976125063612252, 0.9955619646030798, 0.9928826045698136, 0.9895761186026506, 0.9856445951489978, 0.9810905174433342, 0.9759167619387471, 0.9701265964901059, 0.9637236782900092, 0.9567120515588303, 0.9490961449902938, 0.9408807689542252, 0.9320711124582113, 0.9226727398701143, 0.912691587403503, 0.9021339593682022, 0.8910065241883678, 0.8793163101905552, 0.8670707011644898, 0.8542774316992957, 0.8409445822981686, 0.8270805742745622, 0.8126941644330932, 0.7977944395385711, 0.782390810576587, 0.7664930068093497, 0.7501110696304605, 0.7332553462225596, 0.7159364830218318, 0.698165418993472, 0.6799533787224196, 0.6613118653236507, 0.6422526531765844, 0.6227877804881138, 0.6029295416890245, 0.582690479668577, 0.5620833778521299, 0.5411212521268765, 0.5198173426207084, 0.4981851053394912, 0.4762382036679377, 0.45399049973954675, 0.43145604568095713, 0.4086490747363486, 0.38558399227739426, 0.36227536670454485, 0.33873792024528865, 0.31498651965530355, 0.29103616682826866, 0.2669019893203739, 0.2425992307954038, 0.21814324139654043, 0.19354946805085618, 0.16883344471273132, 0.14401078255225114, 0.11909716009486673, 0.09410831331851287, 0.06906002571440237, 0.04396811831786303, 0.01884843971540431, -0.006283143965561256, -0.031410759078129034, -0.056518534482027254, -0.08159061156815871, -0.10661115427526305, -0.1315643590922841, -0.1564344650402344, -0.18120576362713933, -0.20586260876988177, -0.23038942667659296, -0.254770725683383, -0.278991106039232, -0.3030352696327752, -0.32688802965494557, -0.35053432019126063, -0.37395920573780056, -0.39714789063478256, -0.4200857284118068, -0.4427582310389038, -0.46515107807745926, -0.48725012572533494, -0.5090414157503725, -0.5305111843067339, -0.5516458706284317, -0.5724321255945911, -0.5928568201610611, -0.612907053652977, -0.6325701619131265, -0.6518337253008797, -0.6706855765367197, -0.6891138083873496, -0.7071067811865476, -0.724653130187048, -0.7417417727387395, -0.7583619152887234, -0.7745030601987344, -0.79015501237569, -0.8053078857111228, -0.8199521093254521, -0.8340784336131721, -0.8476779360850834, -0.8607420270039448, -0.8732624548099204, -0.8852313113324547, -0.8966410367852363, -0.9074844245411167, -0.9177546256839817, -0.9274451533346613, -0.936549886748193, -0.9450630751798049, -0.9529793415172184, -0.9602936856769433, -0.9670014877624349, -0.9730985109821269, -0.978580904325472, -0.98344520499533, -0.9876883405951378, -0.9913076310695064, -0.9943007903969989, -0.9966659280340298, -0.9984015501089751, -0.9995065603657315, -0.9999802608561371, -0.999822352380809, -0.9990329346781247, -0.9976125063612252, -0.9955619646030798, -0.9928826045698136, -0.9895761186026506, -0.9856445951489978, -0.9810905174433335, -0.9759167619387471, -0.970126596490105, -0.9637236782900093, -0.9567120515588293, -0.9490961449902939, -0.940880768954224, -0.93207111245821, -0.9226727398701144, -0.9126915874035015, -0.9021339593682022, -0.8910065241883662, -0.8793163101905553, -0.8670707011644881, -0.8542774316992939, -0.8409445822981686, -0.8270805742745603, -0.8126941644330933, -0.7977944395385691, -0.7823908105765871, -0.7664930068093475, -0.7501110696304581, -0.7332553462225597, -0.7159364830218294, -0.698165418993472, -0.679953378722417, -0.6613118653236508, -0.6422526531765845, -0.6227877804881111, -0.6029295416890246, -0.5826904796685742, -0.56208337785213, -0.5411212521268737, -0.5198173426207086, -0.4981851053394913, -0.4762382036679378, -0.45399049973954686, -0.43145604568095725, -0.4086490747363487, -0.38558399227739437, -0.36227536670454497, -0.33873792024529215, -0.31498651965530367, -0.2910361668282722, -0.266901989320374, -0.24259923079540738, -0.21814324139654057, -0.1935494680508598, -0.16883344471273493, -0.14401078255225128, -0.11909716009487038, -0.09410831331851299, -0.06906002571440603, -0.043968118317863146, -0.018848439715407984, 0.006283143965557581, 0.03141075907812891, 0.05651853448202358, 0.0815906115681586, 0.1066111542752594, 0.13156435909228395, 0.15643446504023079, 0.18120576362713572, 0.20586260876988163, 0.23038942667658938, 0.2547707256833829, 0.2789911060392285, 0.3030352696327751, 0.3268880296549421, 0.3505343201912605, 0.37395920573780045, 0.39714789063478245, 0.4200857284118067, 0.4427582310389037, 0.46515107807745915, 0.4872501257253348, 0.5090414157503724, 0.5305111843067368, 0.5516458706284317, 0.5724321255945939, 0.592856820161061, 0.6129070536529798, 0.6325701619131264, 0.6518337253008796, 0.6706855765367222, 0.6891138083873495, 0.7071067811865499, 0.7246531301870479, 0.7417417727387419, 0.7583619152887233, 0.7745030601987343, 0.7901550123756921, 0.8053078857111227, 0.8199521093254541, 0.834078433613172, 0.8476779360850851, 0.8607420270039446, 0.8732624548099204, 0.8852313113324564, 0.8966410367852362, 0.9074844245411181, 0.9177546256839817, 0.9274451533346625, 0.936549886748193, 0.9450630751798049, 0.9529793415172194, 0.9602936856769432, 0.9670014877624357, 0.9730985109821267, 0.9785809043254727, 0.98344520499533, 0.9876883405951377, 0.9913076310695068, 0.9943007903969989, 0.9966659280340301, 0.9984015501089751, 0.9995065603657316, 0.9999802608561371, 0.999822352380809, 0.9990329346781247, 0.9976125063612252, 0.9955619646030798, 0.9928826045698136, 0.9895761186026506, 0.9856445951489979, 0.9810905174433342, 0.9759167619387471, 0.9701265964901059, 0.9637236782900093, 0.9567120515588304, 0.9490961449902939, 0.9408807689542253, 0.9320711124582113, 0.9226727398701144, 0.9126915874035031, 0.9021339593682022, 0.8910065241883679, 0.8793163101905553, 0.8670707011644899, 0.8542774316992958, 0.8409445822981687, 0.8270805742745623, 0.8126941644330933, 0.7977944395385713, 0.7823908105765872, 0.7664930068093498, 0.7501110696304606, 0.7332553462225597, 0.715936483021832, 0.6981654189934721, 0.6799533787224198, 0.6613118653236509, 0.6422526531765846, 0.6227877804881112, 0.6029295416890218, 0.5826904796685743, 0.5620833778521273, 0.5411212521268737, 0.5198173426207057, 0.4981851053394883, 0.4762382036679379, 0.4539904997395438, 0.43145604568095736, 0.4086490747363456, 0.3855839922773945, 0.36227536670454175, 0.33873792024528887, 0.3149865196553038, 0.2910361668282689, 0.2669019893203741, 0.24259923079540405, 0.21814324139654068, 0.19354946805085643, 0.16883344471273157, 0.1440107825522514, 0.11909716009486698, 0.09410831331851312, 0.0690600257144026, 0.04396811831786327, 0.018848439715404553, -0.006283143965561011, -0.03141075907812879, -0.05651853448202346, -0.08159061156816201, -0.10661115427526281, -0.13156435909228384, -0.15643446504023065, -0.1812057636271356, -0.205862608769885, -0.23038942667659273, -0.25477072568338277, -0.27899110603922833, -0.3030352696327784, -0.32688802965494534, -0.3505343201912604, -0.37395920573780034, -0.3971478906347791, -0.4200857284118098, -0.4427582310389036, -0.46515107807745903, -0.4872501257253316, -0.5090414157503692, -0.5305111843067367, -0.5516458706284316, -0.5724321255945909, -0.592856820161058, -0.6129070536529797, -0.6325701619131263, -0.6518337253008795, -0.6706855765367196, -0.6891138083873468, -0.7071067811865499, -0.7246531301870478, -0.7417417727387393, -0.758361915288721, -0.7745030601987319, -0.790155012375692, -0.8053078857111226, -0.819952109325452, -0.83407843361317, -0.847677936085085, -0.8607420270039446, -0.8732624548099203, -0.8852313113324546, -0.8966410367852362, -0.9074844245411181, -0.9177546256839816, -0.9274451533346612, -0.936549886748193, -0.9450630751798048, -0.9529793415172194, -0.9602936856769432, -0.9670014877624357, -0.9730985109821267, -0.9785809043254727, -0.98344520499533, -0.9876883405951382, -0.9913076310695068, -0.9943007903969989, -0.9966659280340301, -0.9984015501089752, -0.9995065603657316, -0.9999802608561371, -0.999822352380809, -0.9990329346781245, -0.997612506361225, -0.9955619646030799, -0.9928826045698136, -0.9895761186026502, -0.9856445951489973, -0.9810905174433335, -0.9759167619387471, -0.9701265964901059, -0.9637236782900084, -0.9567120515588294, -0.9490961449902939, -0.9408807689542253, -0.9320711124582114, -0.9226727398701131, -0.9126915874035016, -0.9021339593682023, -0.891006524188368, -0.8793163101905538, -0.8670707011644883, -0.854277431699294, -0.8409445822981688, -0.8270805742745624, -0.8126941644330913, -0.7977944395385692, -0.7823908105765872, -0.76649300680935, -0.7501110696304607, -0.7332553462225574, -0.7159364830218296, -0.6981654189934722, -0.6799533787224198, -0.6613118653236484, -0.642252653176582, -0.6227877804881113, -0.6029295416890247, -0.5826904796685773, -0.5620833778521274, -0.5411212521268738, -0.5198173426207088, -0.49818510533949145, -0.4762382036679411, -0.4539904997395439, -0.43145604568095747, -0.4086490747363489, -0.38558399227739787, -0.3622753667045485, -0.33873792024528904, -0.3149865196553039, -0.29103616682827244, -0.2669019893203777, -0.24259923079540416, -0.2181432413965408, -0.19354946805086, -0.16883344471273518, -0.14401078255225502, -0.11909716009486711, -0.09410831331851323, -0.06906002571440627, -0.04396811831786694, -0.018848439715408227, 0.006283143965560888, 0.03141075907812867, 0.056518534482026886, 0.08159061156815835, 0.10661115427526269, 0.13156435909228373, 0.15643446504023403, 0.18120576362713897, 0.2058626087698814, 0.2303894266765926, 0.2547707256833861, 0.27899110603923166, 0.3030352696327749, 0.3268880296549419, 0.3505343201912636, 0.37395920573780356, 0.39714789063478223, 0.42008572841180647, 0.44275823103890666, 0.46515107807746203, 0.4872501257253346, 0.5090414157503722, 0.5305111843067336, 0.5516458706284315, 0.5724321255945908, 0.5928568201610579, 0.6129070536529739, 0.6325701619131208, 0.6518337253008794, 0.6706855765367195, 0.6891138083873467, 0.7071067811865448, 0.7246531301870478, 0.7417417727387392, 0.7583619152887209, 0.7745030601987318, 0.7901550123756875, 0.8053078857111224, 0.8199521093254519, 0.8340784336131699, 0.8476779360850812, 0.8607420270039409, 0.8732624548099203, 0.8852313113324546, 0.8966410367852345, 0.907484424541115, 0.9177546256839816, 0.9274451533346612, 0.9365498867481916, 0.9450630751798036, 0.9529793415172172, 0.9602936856769432, 0.9670014877624348, 0.973098510982126, 0.9785809043254712, 0.9834452049953286, 0.9876883405951377, 0.9913076310695063, 0.9943007903969985, 0.9966659280340294, 0.998401550108975, 0.9995065603657315, 0.9999802608561371, 0.9998223523808091, 0.999032934678125, 0.9976125063612252, 0.9955619646030802, 0.992882604569814, 0.9895761186026517, 0.9856445951489992, 0.9810905174433343, 0.975916761938748, 0.9701265964901068, 0.9637236782900113, 0.9567120515588305, 0.9490961449902952, 0.9408807689542266, 0.9320711124582127, 0.9226727398701173, 0.9126915874035032, 0.9021339593682038, 0.8910065241883697, 0.8793163101905589, 0.8670707011644936, 0.8542774316992959, 0.8409445822981707, 0.8270805742745645, 0.8126941644330976, 0.7977944395385714, 0.7823908105765895, 0.7664930068093523, 0.7501110696304631, 0.7332553462225647, 0.7159364830218322, 0.6981654189934748, 0.6799533787224226, 0.6613118653236565, 0.6422526531765903, 0.6227877804881142, 0.6029295416890277, 0.5826904796685803, 0.5620833778521362, 0.5411212521268769, 0.5198173426207119, 0.49818510533949467, 0.4762382036679444, 0.4539904997395535, 0.4314560456809608, 0.4086490747363523, 0.38558399227740126, 0.3622753667045519, 0.33873792024529914, 0.3149865196553074, 0.29103616682827593, 0.2669019893203812, 0.24259923079541462, 0.21814324139654437, 0.19354946805086362, 0.1688334447127388, 0.14401078255225866, 0.11909716009487076, 0.09410831331851689, 0.06906002571440994, 0.043968118317863514, 0.01884843971540835, -0.006283143965557213, -0.031410759078124996, -0.05651853448202676, -0.08159061156815822, -0.10661115427525902, -0.13156435909228006, -0.15643446504023392, -0.18120576362713886, -0.20586260876988127, -0.23038942667658902, -0.254770725683386, -0.27899110603923155, -0.3030352696327747, -0.32688802965494174, -0.35053432019125685, -0.37395920573780345, -0.3971478906347821, -0.42008572841180636, -0.4427582310389002, -0.4651510780774619, -0.4872501257253345, -0.5090414157503721, -0.5305111843067335, -0.5516458706284284, -0.5724321255945937, -0.5928568201610607, -0.6129070536529767, -0.6325701619131234, -0.6518337253008766, -0.670685576536722, -0.6891138083873493, -0.7071067811865471, -0.7246531301870452, -0.7417417727387368, -0.7583619152887231, -0.774503060198734, -0.7901550123756896, -0.8053078857111203, -0.8199521093254539, -0.8340784336131719, -0.847677936085083, -0.8607420270039426, -0.8732624548099185, -0.8852313113324561, -0.8966410367852361, -0.9074844245411164, -0.9177546256839801, -0.9274451533346597, -0.9365498867481928, -0.9450630751798048, -0.9529793415172183, -0.9602936856769422, -0.9670014877624357, -0.9730985109821267, -0.978580904325472, -0.9834452049953293, -0.9876883405951371, -0.9913076310695068, -0.9943007903969989, -0.9966659280340298, -0.9984015501089749, -0.9995065603657314, -0.9999802608561371, -0.9998223523808091, -0.9990329346781248, -0.9976125063612254, -0.9955619646030799, -0.9928826045698137, -0.9895761186026512, -0.9856445951489986, -0.981090517443335, -0.9759167619387472, -0.970126596490106, -0.9637236782900103, -0.9567120515588315, -0.9490961449902963, -0.9408807689542255, -0.9320711124582115, -0.922672739870116, -0.9126915874035046, -0.9021339593682024, -0.8910065241883681, -0.8793163101905572, -0.8670707011644919, -0.8542774316992979, -0.8409445822981689, -0.8270805742745625, -0.8126941644330956, -0.7977944395385737, -0.7823908105765918, -0.7664930068093501, -0.7501110696304608, -0.7332553462225624, -0.7159364830218348, -0.6981654189934724, -0.67995337872242, -0.6613118653236539, -0.6422526531765876, -0.622787780488117, -0.6029295416890249, -0.5826904796685776, -0.5620833778521334, -0.54112125212688, -0.5198173426207151, -0.4981851053394917, -0.47623820366794134, -0.45399049973955047, -0.43145604568096413, -0.40864907473634915, -0.3855839922773981, -0.36227536670454874, -0.3387379202452959, -0.3149865196553109, -0.29103616682827266, -0.2669019893203779, -0.2425992307954113, -0.21814324139654798, -0.19354946805086723, -0.16883344471273543, -0.14401078255225527, -0.11909716009487441, -0.09410831331852056, -0.06906002571440652, -0.043968118317867184, -0.018848439715412026, 0.006283143965553538, 0.03141075907812132, 0.05651853448202309, 0.08159061156815456, 0.10661115427525537, 0.13156435909227643, 0.15643446504022326, 0.18120576362713525, 0.2058626087698777, 0.23038942667658546, 0.25477072568337555, 0.278991106039228, 0.3030352696327712, 0.3268880296549383, 0.3505343201912534, 0.3739592057377934, 0.3971478906347788, 0.420085728411803, 0.4427582310388969, 0.46515107807745243, 0.4872501257253251, 0.509041415750369, 0.5305111843067304, 0.5516458706284253, 0.5724321255945848, 0.5928568201610577, 0.6129070536529737, 0.6325701619131205, 0.6518337253008791, 0.6706855765367192, 0.6891138083873466, 0.7071067811865446, 0.7246531301870476, 0.7417417727387391, 0.7583619152887207, 0.7745030601987317, 0.7901550123756917, 0.8053078857111223, 0.8199521093254518, 0.8340784336131698, 0.8476779360850849, 0.8607420270039444, 0.8732624548099202, 0.8852313113324545, 0.8966410367852375, 0.9074844245411179, 0.9177546256839815, 0.927445153334661, 0.9365498867481915, 0.9450630751798059, 0.9529793415172193, 0.9602936856769431, 0.9670014877624347, 0.9730985109821275, 0.9785809043254726, 0.9834452049953298, 0.9876883405951377, 0.9913076310695063, 0.9943007903969993, 0.99666592803403, 0.998401550108975, 0.9995065603657315, 0.9999802608561371, 0.999822352380809, 0.9990329346781247, 0.9976125063612252, 0.9955619646030802, 0.9928826045698141, 0.9895761186026507, 0.9856445951489979, 0.9810905174433343, 0.975916761938748, 0.9701265964901051, 0.9637236782900094, 0.9567120515588305, 0.9490961449902952, 0.9408807689542267, 0.9320711124582102, 0.9226727398701147, 0.9126915874035032, 0.902133959368204, 0.8910065241883698, 0.8793163101905556, 0.8670707011644901, 0.8542774316992962, 0.8409445822981709, 0.8270805742745606, 0.8126941644330936, 0.7977944395385715, 0.7823908105765897, 0.7664930068093525, 0.7501110696304586, 0.7332553462225601, 0.7159364830218323, 0.698165418993475, 0.6799533787224227, 0.6613118653236513, 0.642252653176585, 0.6227877804881143, 0.6029295416890279, 0.5826904796685748, 0.5620833778521306, 0.5411212521268771, 0.5198173426207121, 0.4981851053394949, 0.47623820366793834, 0.4539904997395474, 0.431456045680961, 0.40864907473635254, 0.38558399227740153, 0.3622753667045455, 0.3387379202452927, 0.3149865196553076, 0.29103616682827615, 0.26690198932037457, 0.24259923079540796, 0.21814324139654462, 0.19354946805086387, 0.16883344471273903, 0.14401078255225186, 0.119097160094871, 0.09410831331851714, 0.06906002571441018, 0.043968118317870855, 0.018848439715408595, -0.006283143965556968, -0.031410759078124746, -0.05651853448201942, -0.08159061156815799, -0.10661115427525879, -0.13156435909227984, -0.15643446504022665, -0.18120576362713162, -0.20586260876988105, -0.2303894266765888, -0.2547707256833789, -0.27899110603922445, -0.3030352696327677, -0.3268880296549415, -0.35053432019125663, -0.3739592057377966, -0.3971478906347754, -0.42008572841180614, -0.4427582310389, -0.4651510780774554, -0.4872501257253281, -0.5090414157503658, -0.5305111843067333, -0.5516458706284282, -0.5724321255945876, -0.5928568201610548, -0.6129070536529708, -0.6325701619131232, -0.6518337253008764, -0.6706855765367166, -0.6891138083873439, -0.707106781186547, -0.724653130187045, -0.7417417727387366, -0.7583619152887183, -0.7745030601987294, -0.7901550123756894, -0.8053078857111202, -0.8199521093254497, -0.8340784336131678, -0.8476779360850791, -0.8607420270039425, -0.8732624548099184, -0.8852313113324527, -0.8966410367852328, -0.9074844245411163, -0.91775462568398, -0.9274451533346597, -0.9365498867481903, -0.9450630751798024, -0.9529793415172182, -0.9602936856769421, -0.9670014877624338, -0.973098510982125, -0.9785809043254718, -0.9834452049953292, -0.9876883405951371, -0.9913076310695058, -0.9943007903969988, -0.9966659280340298, -0.9984015501089748, -0.9995065603657314, -0.9999802608561371, -0.9998223523808091, -0.9990329346781248, -0.9976125063612254, -0.9955619646030799, -0.9928826045698137, -0.9895761186026513, -0.9856445951489986, -0.9810905174433336, -0.9759167619387472, -0.970126596490106, -0.9637236782900104, -0.9567120515588295, -0.9490961449902942, -0.9408807689542255, -0.9320711124582115, -0.9226727398701133, -0.9126915874035019, -0.9021339593682025, -0.8910065241883682, -0.8793163101905573, -0.8670707011644885, -0.8542774316992944, -0.840944582298169, -0.8270805742745626, -0.8126941644330916, -0.7977944395385695, -0.7823908105765875, -0.7664930068093503, -0.750111069630461, -0.7332553462225577, -0.7159364830218299, -0.6981654189934725, -0.6799533787224202, -0.661311865323654, -0.6422526531765824, -0.6227877804881117, -0.6029295416890251, -0.5826904796685778, -0.5620833778521277, -0.5411212521268742, -0.5198173426207092, -0.4981851053394919, -0.47623820366794156, -0.45399049973954436, -0.4314560456809579, -0.40864907473634937, -0.38558399227739837, -0.36227536670454896, -0.3387379202452895, -0.31498651965530433, -0.2910361668282729, -0.2669019893203781, -0.24259923079541154, -0.21814324139654126, -0.1935494680508605, -0.16883344471273568, -0.1440107825522555, -0.1190971600948676, -0.09410831331851373, -0.06906002571440677, -0.043968118317867434, -0.01884843971541227, 0.006283143965560399, 0.031410759078128174, 0.05651853448202285, 0.08159061156815432, 0.10661115427525514, 0.13156435909228323, 0.15643446504023004, 0.181205763627135, 0.20586260876987744, 0.23038942667659212, 0.2547707256833822, 0.2789911060392278, 0.303035269632771, 0.3268880296549381, 0.3505343201912598, 0.3739592057377998, 0.3971478906347785, 0.4200857284118028, 0.44275823103889667, 0.4651510780774585, 0.4872501257253311, 0.5090414157503688, 0.5305111843067302, 0.5516458706284311, 0.5724321255945904, 0.5928568201610576, 0.6129070536529736, 0.6325701619131204, 0.651833725300879, 0.6706855765367191, 0.6891138083873464, 0.7071067811865444, 0.7246531301870426, 0.7417417727387389, 0.7583619152887205, 0.7745030601987316, 0.7901550123756872, 0.8053078857111222, 0.8199521093254517, 0.8340784336131697, 0.847677936085081, 0.8607420270039406, 0.87326245480992, 0.8852313113324544, 0.8966410367852343, 0.9074844245411149, 0.9177546256839786, 0.9274451533346609, 0.9365498867481914, 0.9450630751798035, 0.9529793415172171, 0.9602936856769431, 0.9670014877624347, 0.9730985109821259, 0.9785809043254711, 0.9834452049953285, 0.9876883405951375, 0.9913076310695063, 0.9943007903969985, 0.9966659280340294, 0.9984015501089747, 0.9995065603657315, 0.9999802608561371, 0.9998223523808091, 0.999032934678125, 0.9976125063612252, 0.9955619646030802, 0.9928826045698141, 0.9895761186026517, 0.9856445951489993, 0.9810905174433344, 0.9759167619387481, 0.9701265964901069, 0.9637236782900114, 0.9567120515588328, 0.9490961449902953, 0.9408807689542268, 0.9320711124582128, 0.9226727398701174, 0.9126915874035033, 0.9021339593682041, 0.8910065241883699, 0.8793163101905591, 0.8670707011644938, 0.8542774316992963, 0.840944582298171, 0.8270805742745647, 0.8126941644330978, 0.7977944395385718, 0.7823908105765899, 0.7664930068093526, 0.7501110696304635, 0.7332553462225603, 0.7159364830218325, 0.6981654189934752, 0.6799533787224229, 0.6613118653236515, 0.6422526531765852, 0.6227877804881146, 0.602929541689028, 0.582690479668575, 0.5620833778521308, 0.5411212521268773, 0.5198173426207123, 0.49818510533948895, 0.47623820366793856, 0.45399049973954764, 0.43145604568096124, 0.40864907473634626, 0.38558399227739515, 0.36227536670454574, 0.3387379202452929, 0.3149865196553011, 0.2910361668282696, 0.26690198932037484, 0.2425992307954082, 0.21814324139654487, 0.19354946805085715, 0.1688334447127323, 0.1440107825522521, 0.11909716009487124, 0.09410831331851031, 0.06906002571440334, 0.043968118317864006, 0.01884843971540884, -0.006283143965556724, -0.03141075907813161, -0.056518534482026275, -0.08159061156815774, -0.10661115427525854, -0.1315643590922796, -0.15643446504023342, -0.18120576362713836, -0.2058626087698808, -0.23038942667658854, -0.2547707256833855, -0.27899110603923105, -0.3030352696327743, -0.3268880296549413, -0.35053432019125635, -0.37395920573780295, -0.3971478906347817, -0.4200857284118059, -0.4427582310388998, -0.4651510780774552, -0.48725012572533405, -0.5090414157503717, -0.530511184306733, -0.551645870628428, -0.5724321255945932, -0.5928568201610603, -0.6129070536529763, -0.632570161913123, -0.6518337253008761, -0.6706855765367217, -0.6891138083873489, -0.7071067811865468, -0.7246531301870449, -0.7417417727387364, -0.7583619152887228, -0.7745030601987337, -0.7901550123756893, -0.80530788571112, -0.8199521093254496, -0.8340784336131716, -0.8476779360850828, -0.8607420270039424, -0.8732624548099183, -0.8852313113324559, -0.8966410367852359, -0.9074844245411162, -0.9177546256839799, -0.9274451533346596, -0.9365498867481926, -0.9450630751798046, -0.9529793415172181, -0.960293685676942, -0.9670014877624337, -0.9730985109821266, -0.9785809043254718, -0.9834452049953292, -0.987688340595137, -0.9913076310695067, -0.9943007903969988, -0.9966659280340298, -0.9984015501089748, -0.9995065603657314, -0.9999802608561371, -0.9998223523808091, -0.9990329346781248, -0.9976125063612256, -0.9955619646030806, -0.9928826045698137, -0.9895761186026513, -0.9856445951489986, -0.9810905174433351, -0.9759167619387473, -0.9701265964901061, -0.9637236782900105, -0.9567120515588318, -0.9490961449902965, -0.9408807689542256, -0.9320711124582116, -0.9226727398701162, -0.9126915874035049, -0.9021339593682056, -0.8910065241883683, -0.8793163101905574, -0.8670707011644921, -0.8542774316992982, -0.8409445822981692, -0.8270805742745628, -0.8126941644330958, -0.7977944395385739, -0.7823908105765921, -0.7664930068093504, -0.7501110696304611, -0.7332553462225627, -0.7159364830218351, -0.6981654189934778, -0.6799533787224203, -0.6613118653236543, -0.642252653176588, -0.6227877804881174, -0.6029295416890254, -0.5826904796685779, -0.5620833778521338, -0.5411212521268804, -0.5198173426207154, -0.4981851053394921, -0.4762382036679418, -0.4539904997395509, -0.4314560456809645, -0.4086490747363561, -0.3855839922773986, -0.3622753667045492, -0.33873792024529636, -0.3149865196553113, -0.2910361668282731, -0.26690198932037834, -0.24259923079541176, -0.21814324139654845, -0.19354946805086773, -0.1688334447127359, -0.14401078255225574, -0.1190971600948749, -0.09410831331852104, -0.069060025714407, -0.04396811831786768, -0.018848439715412516, 0.006283143965553048, 0.03141075907812793, 0.056518534482022605, 0.08159061156815407, 0.10661115427525489, 0.13156435909228298, 0.15643446504022981, 0.18120576362713475, 0.20586260876987722, 0.23038942667659187, 0.25477072568338194, 0.27899110603922755, 0.30303526963277755, 0.3268880296549445, 0.3505343201912596, 0.37395920573779956, 0.39714789063478484, 0.420085728411809, 0.4427582310389028, 0.46515107807745826, 0.4872501257253309, 0.5090414157503746, 0.530511184306736, 0.5516458706284308, 0.5724321255945902, 0.5928568201610573, 0.612907053652979, 0.6325701619131257, 0.6518337253008788, 0.6706855765367189, 0.6891138083873514, 0.7071067811865492, 0.7246531301870472, 0.7417417727387388, 0.7583619152887204, 0.7745030601987359, 0.7901550123756914, 0.805307885711122, 0.8199521093254516, 0.8340784336131696, 0.8476779360850846, 0.8607420270039442, 0.8732624548099199, 0.8852313113324543, 0.8966410367852374, 0.9074844245411178, 0.9177546256839813, 0.9274451533346608, 0.9365498867481914, 0.9450630751798057, 0.9529793415172192, 0.960293685676943, 0.9670014877624346, 0.9730985109821257, 0.9785809043254725, 0.9834452049953297, 0.9876883405951375, 0.9913076310695063, 0.9943007903969991, 0.99666592803403, 0.998401550108975, 0.9995065603657315, 0.9999802608561371, 0.999822352380809, 0.9990329346781247, 0.9976125063612252, 0.9955619646030802, 0.9928826045698141, 0.9895761186026508, 0.985644595148998, 0.9810905174433344, 0.9759167619387481, 0.9701265964901052, 0.9637236782900095, 0.9567120515588308, 0.9490961449902954, 0.9408807689542268, 0.9320711124582104, 0.9226727398701149, 0.9126915874035034, 0.9021339593682042, 0.89100652418837, 0.8793163101905559, 0.8670707011644905, 0.8542774316992964, 0.8409445822981712, 0.8270805742745648, 0.8126941644330938, 0.7977944395385719, 0.78239081057659, 0.7664930068093527, 0.7501110696304589, 0.7332553462225604, 0.7159364830218327, 0.6981654189934753, 0.679953378722423, 0.6613118653236517, 0.6422526531765854, 0.6227877804881148, 0.6029295416890282, 0.5826904796685809, 0.562083377852131, 0.5411212521268776, 0.5198173426207126, 0.4981851053394953, 0.4762382036679388, 0.45399049973954786, 0.43145604568096146, 0.408649074736353, 0.385583992277402, 0.36227536670454596, 0.33873792024529314, 0.31498651965530805, 0.29103616682827665, 0.2669019893203819, 0.24259923079540843, 0.2181432413965451, 0.19354946805086434, 0.16883344471273953, 0.14401078255225236, 0.11909716009487148, 0.09410831331851763, 0.06906002571441067, 0.04396811831787135, 0.018848439715409084, -0.006283143965556478, -0.03141075907812426, -0.056518534482018934, -0.08159061156815041, -0.1066111542752583, -0.13156435909227934, -0.15643446504022618, -0.18120576362713114, -0.20586260876988055, -0.23038942667658832, -0.2547707256833784, -0.278991106039224, -0.3030352696327673, -0.32688802965494107, -0.35053432019125613, -0.3739592057377962, -0.39714789063477496, -0.4200857284117992, -0.44275823103889955, -0.46515107807745504, -0.48725012572532767, -0.5090414157503653, -0.5305111843067329, -0.5516458706284277, -0.5724321255945872, -0.5928568201610543, -0.6129070536529705, -0.6325701619131229, -0.651833725300876, -0.6706855765367161, -0.6891138083873436, -0.7071067811865467, -0.7246531301870447, -0.7417417727387363, -0.758361915288718, -0.7745030601987336, -0.7901550123756892, -0.8053078857111199, -0.8199521093254494, -0.8340784336131715, -0.8476779360850827, -0.8607420270039423, -0.8732624548099216, -0.8852313113324558, -0.8966410367852358, -0.9074844245411162, -0.9177546256839826, -0.9274451533346622, -0.9365498867481925, -0.9450630751798045, -0.9529793415172202, -0.960293685676944, -0.9670014877624354, -0.9730985109821265, -0.9785809043254717, -0.9834452049953304, -0.9876883405951381, -0.9913076310695067, -0.9943007903969988, -0.9966659280340296, -0.9984015501089752, -0.9995065603657316, -0.9999802608561371, -0.9998223523808091, -0.9990329346781246, -0.997612506361225, -0.9955619646030799, -0.9928826045698137, -0.9895761186026513, -0.9856445951489975, -0.9810905174433338, -0.9759167619387473, -0.9701265964901061, -0.9637236782900105, -0.9567120515588298, -0.9490961449902943, -0.9408807689542257, -0.9320711124582117, -0.9226727398701136, -0.9126915874035021, -0.9021339593682027, -0.8910065241883685, -0.8793163101905576, -0.8670707011644887, -0.8542774316992946, -0.8409445822981693, -0.8270805742745629, -0.8126941644330961, -0.7977944395385698, -0.7823908105765879, -0.7664930068093505, -0.7501110696304614, -0.7332553462225581, -0.7159364830218302, -0.6981654189934728, -0.6799533787224153, -0.6613118653236545, -0.6422526531765828, -0.6227877804881177, -0.6029295416890255, -0.5826904796685723, -0.562083377852134, -0.5411212521268747, -0.5198173426207157, -0.49818510533949234, -0.47623820366793573, -0.45399049973955113, -0.43145604568095836, -0.4086490747363563, -0.3855839922773988, -0.3622753667045428, -0.33873792024529664, -0.31498651965530483, -0.29103616682826655, -0.2669019893203786, -0.2425992307954051, -0.21814324139654867, -0.19354946805086098, -0.16883344471272915, -0.144010782552256, -0.11909716009486808, -0.09410831331852128, -0.06906002571440725, -0.04396811831786082, -0.01884843971541276, 0.006283143965559909, 0.03141075907812058, 0.05651853448202236, 0.08159061156816091, 0.10661115427525464, 0.13156435909228276, 0.15643446504022254, 0.18120576362713453, 0.2058626087698839, 0.23038942667658474, 0.2547707256833817, 0.27899110603922045, 0.30303526963277055, 0.3268880296549443, 0.3505343201912527, 0.37395920573779934, 0.39714789063477157, 0.42008572841180236, 0.4427582310389026, 0.46515107807745176, 0.48725012572533066, 0.5090414157503744, 0.5305111843067298, 0.5516458706284306, 0.5724321255945842, 0.5928568201610571, 0.6129070536529788, 0.63257016191312, 0.6518337253008786, 0.6706855765367135, 0.689113808387346, 0.707106781186549, 0.7246531301870422, 0.7417417727387385, 0.7583619152887155, 0.7745030601987313, 0.7901550123756913, 0.8053078857111177, 0.8199521093254514, 0.8340784336131655, 0.8476779360850807, 0.8607420270039441, 0.8732624548099164, 0.8852313113324541, 0.896641036785231, 0.9074844245411147, 0.9177546256839811, 0.927445153334658, 0.9365498867481913, 0.9450630751798056, 0.952979341517217, 0.9602936856769428, 0.9670014877624327, 0.9730985109821257, 0.9785809043254725, 0.9834452049953284, 0.9876883405951375, 0.9913076310695061, 0.9943007903969984, 0.99666592803403, 0.9984015501089746, 0.9995065603657315, 0.9999802608561371, 0.9998223523808091, 0.9990329346781247, 0.9976125063612253, 0.9955619646030803, 0.9928826045698141, 0.9895761186026508, 0.985644595148998, 0.9810905174433344, 0.9759167619387482, 0.9701265964901071, 0.9637236782900096, 0.9567120515588308, 0.9490961449902954, 0.9408807689542245, 0.9320711124582105, 0.9226727398701149, 0.9126915874035035, 0.9021339593682043, 0.8910065241883669, 0.879316310190556, 0.8670707011644906, 0.8542774316992928, 0.8409445822981713, 0.827080574274561, 0.8126941644330941, 0.797794439538572, 0.7823908105765858, 0.766493006809353, 0.750111069630459, 0.7332553462225557, 0.7159364830218329, 0.6981654189934704, 0.6799533787224232, 0.6613118653236518, 0.6422526531765801, 0.622787780488115, 0.6029295416890228, 0.5826904796685811, 0.5620833778521311, 0.5411212521268718, 0.5198173426207128, 0.49818510533948934, 0.47623820366793274, 0.4539904997395481, 0.43145604568095525, 0.4086490747363532, 0.38558399227739565, 0.3622753667045396, 0.33873792024529337, 0.31498651965530156, 0.2910361668282769, 0.2669019893203753, 0.24259923079540177, 0.21814324139654534, 0.19354946805085763, 0.16883344471273976, 0.1440107825522526, 0.11909716009486467, 0.09410831331851786, 0.06906002571440382, 0.04396811831787159, 0.01884843971540933, -0.006283143965563339, -0.03141075907812401, -0.05651853448202578, -0.08159061156815017, -0.10661115427525805, -0.13156435909228614, -0.15643446504022593, -0.1812057636271379, -0.20586260876988727, -0.23038942667658807, -0.25477072568338505, -0.2789911060392238, -0.30303526963277383, -0.32688802965494757, -0.3505343201912559, -0.3739592057378025, -0.39714789063477474, -0.42008572841180547, -0.4427582310389057, -0.4651510780774548, -0.48725012572533366, -0.5090414157503651, -0.5305111843067327, -0.5516458706284335, -0.572432125594587, -0.5928568201610599, -0.6129070536529703, -0.6325701619131227, -0.6518337253008812, -0.670685576536716, -0.6891138083873485, -0.7071067811865415, -0.7246531301870446, -0.7417417727387409, -0.7583619152887179, -0.7745030601987334, -0.7901550123756934, -0.8053078857111198, -0.8199521093254534, -0.8340784336131674, -0.8476779360850826, -0.8607420270039458, -0.873262454809918, -0.8852313113324557, -0.8966410367852325, -0.9074844245411161, -0.9177546256839826, -0.9274451533346594, -0.9365498867481925, -0.9450630751798021, -0.952979341517218, -0.9602936856769438, -0.9670014877624336, -0.9730985109821265, -0.9785809043254703, -0.9834452049953291, -0.9876883405951381, -0.9913076310695057, -0.9943007903969988, -0.9966659280340291, -0.9984015501089748, -0.9995065603657316, -0.9999802608561371, -0.9998223523808091, -0.9990329346781252, -0.9976125063612256, -0.99556196460308, -0.9928826045698146, -0.9895761186026514, -0.9856445951489975, -0.9810905174433352, -0.9759167619387474, -0.970126596490108, -0.9637236782900106, -0.9567120515588298, -0.9490961449902966, -0.9408807689542258, -0.9320711124582144, -0.9226727398701163, -0.9126915874035022, -0.9021339593682058, -0.8910065241883686, -0.8793163101905611, -0.8670707011644924, -0.8542774316992947, -0.8409445822981733, -0.827080574274563, -0.8126941644330962, -0.7977944395385742, -0.782390810576588, -0.7664930068093553, -0.7501110696304615, -0.733255346222563, -0.7159364830218354, -0.6981654189934731, -0.6799533787224208, -0.6613118653236546, -0.642252653176583, -0.6227877804881122, -0.6029295416890257, -0.5826904796685783, -0.5620833778521342, -0.5411212521268749, -0.5198173426207098, -0.49818510533949256, -0.47623820366794223, -0.453990499739545, -0.4314560456809586, -0.4086490747363501, -0.38558399227739903, -0.36227536670454963, -0.33873792024529015, -0.31498651965530505, -0.2910361668282736, -0.266901989320372, -0.24259923079541224, -0.21814324139654198, -0.19354946805086123, -0.1688334447127364, -0.1440107825522492, -0.11909716009487538, -0.09410831331851445, -0.06906002571440041, -0.04396811831786816, -0.0188484397154059, 0.006283143965566769, 0.031410759078127445, 0.05651853448202921, 0.08159061156815359, 0.10661115427526147, 0.13156435909228956, 0.15643446504022931, 0.18120576362714128, 0.20586260876987672, 0.2303894266765914, 0.2547707256833883, 0.27899110603922705, 0.3030352696327771, 0.32688802965493735, 0.35053432019125913, 0.3739592057378057, 0.39714789063477784, 0.4200857284118086, 0.44275823103889606, 0.4651510780774578, 0.48725012572533666, 0.5090414157503681, 0.5305111843067356, 0.5516458706284245, 0.5724321255945898, 0.5928568201610627, 0.612907053652973, 0.6325701619131253, 0.6518337253008838, 0.6706855765367186, 0.689113808387351, 0.7071067811865439, 0.7246531301870469, 0.7417417727387432, 0.7583619152887201, 0.7745030601987356, 0.7901550123756867, 0.8053078857111218, 0.8199521093254553, 0.8340784336131692, 0.8476779360850843, 0.8607420270039403, 0.8732624548099197, 0.8852313113324572, 0.896641036785234, 0.9074844245411176, 0.9177546256839783, 0.9274451533346607, 0.9365498867481962, 0.9450630751798033, 0.9529793415172212, 0.9602936856769408, 0.9670014877624362, 0.9730985109821273, 0.9785809043254724, 0.9834452049953297, 0.9876883405951397, 0.9913076310695061, 0.9943007903969999, 0.9966659280340293, 0.9984015501089754, 0.9995065603657317, 0.9999802608561371, 0.999822352380809, 0.9990329346781247, 0.9976125063612253, 0.995561964603079, 0.9928826045698143, 0.9895761186026498, 0.9856445951489994, 0.9810905174433331, 0.9759167619387467, 0.9701265964901055, 0.9637236782900096, 0.9567120515588309, 0.9490961449902955, 0.9408807689542221, 0.9320711124582132, 0.9226727398701123, 0.9126915874035065, 0.9021339593682013, 0.891006524188367, 0.8793163101905561, 0.8670707011644907, 0.8542774316992893, 0.8409445822981714, 0.8270805742745572, 0.8126941644330983, 0.7977944395385679, 0.7823908105765859, 0.7664930068093485, 0.7501110696304593, 0.7332553462225607, 0.715936483021833, 0.6981654189934655, 0.6799533787224235, 0.6613118653236467, 0.6422526531765912, 0.6227877804881096, 0.602929541689023, 0.5826904796685756, 0.5620833778521314, 0.541121252126878, 0.519817342620713, 0.4981851053394834, 0.47623820366794545, 0.4539904997395419, 0.4314560456809683, 0.40864907473634693, 0.38558399227739587, 0.36227536670454646, 0.33873792024529364, 0.31498651965530855, 0.2910361668282771, 0.2669019893203687, 0.24259923079541582, 0.21814324139653865, 0.19354946805085788, 0.168833444712733, 0.14401078255225283, 0.11909716009487196, 0.09410831331851811, 0.06906002571439698, 0.04396811831787184, 0.01884843971540247, -0.006283143965548884, -0.03141075907813087, -0.05651853448202554, -0.081590611568157, -0.10661115427525782, -0.13156435909227887, -0.15643446504022568, -0.18120576362714463, -0.20586260876987314, -0.23038942667659476, -0.25477072568337106, -0.27899110603923033, -0.30303526963277355, -0.3268880296549406, -0.3505343201912557, -0.3739592057377957, -0.3971478906347745, -0.4200857284118117, -0.4427582310388927, -0.46515107807746087, -0.48725012572533344, -0.5090414157503711, -0.5305111843067325, -0.5516458706284274, -0.5724321255945868, -0.5928568201610654, -0.61290705365297, -0.632570161913128, -0.6518337253008702, -0.6706855765367211, -0.6891138083873484, -0.7071067811865464, -0.7246531301870444, -0.741741772738736, -0.7583619152887177, -0.7745030601987377, -0.7901550123756845, -0.8053078857111238, -0.819952109325445, -0.8340784336131711, -0.8476779360850824, -0.8607420270039421, -0.8732624548099179, -0.8852313113324523, -0.8966410367852324, -0.907484424541119, -0.9177546256839768, -0.9274451533346619, -0.9365498867481924, -0.9450630751798044, -0.9529793415172179, -0.9602936856769418, -0.9670014877624334, -0.9730985109821281, -0.9785809043254702, -0.9834452049953303, -0.9876883405951358, -0.9913076310695066, -0.9943007903969987, -0.9966659280340296, -0.9984015501089748, -0.9995065603657314, -0.9999802608561371, -0.999822352380809, -0.9990329346781252, -0.9976125063612251, -0.9955619646030813, -0.9928826045698138, -0.9895761186026514, -0.9856445951489987, -0.9810905174433352, -0.975916761938749, -0.970126596490108, -0.9637236782900087, -0.956712051558834, -0.9490961449902944, -0.9408807689542258, -0.932071112458212, -0.9226727398701164, -0.9126915874035052, -0.902133959368206, -0.8910065241883655, -0.8793163101905612, -0.8670707011644889, -0.8542774316992948, -0.8409445822981696, -0.8270805742745633, -0.8126941644330963, -0.7977944395385743, -0.7823908105765925, -0.7664930068093463, -0.7501110696304569, -0.7332553462225584, -0.7159364830218307, -0.6981654189934732, -0.6799533787224209, -0.6613118653236548, -0.6422526531765885, -0.6227877804881069, -0.6029295416890316, -0.5826904796685728, -0.5620833778521286, -0.541121252126875, -0.51981734262071, -0.49818510533949273, -0.47623820366794245, -0.45399049973953887, -0.4314560456809652, -0.4086490747363438, -0.3855839922773927, -0.36227536670454324, -0.33873792024529037, -0.3149865196553053, -0.2910361668282738, -0.26690198932036535, -0.24259923079541248, -0.2181432413965353, -0.19354946805086845, -0.16883344471272962, -0.14401078255224944, -0.11909716009486856, -0.0941083133185147, -0.06906002571440774, -0.04396811831786841, -0.01884843971539904, 0.006283143965552313, 0.0314107590781343, 0.05651853448201478, 0.08159061156816043, 0.10661115427526122, 0.13156435909228226, 0.1564344650402291, 0.18120576362714802, 0.2058626087698765, 0.2303894266765981, 0.2547707256833744, 0.27899110603923366, 0.3030352696327768, 0.32688802965494385, 0.3505343201912589, 0.3739592057377989, 0.3971478906347776, 0.4200857284118148, 0.44275823103889583, 0.4651510780774639, 0.487250125725324, 0.509041415750374, 0.5305111843067354, 0.5516458706284303, 0.5724321255945897, 0.5928568201610568, 0.6129070536529728, 0.6325701619131306, 0.6518337253008728, 0.6706855765367237, 0.6891138083873405, 0.7071067811865488, 0.7246531301870467, 0.7417417727387383, 0.7583619152887199, 0.7745030601987309, 0.7901550123756866, 0.8053078857111259, 0.819952109325447, 0.834078433613173, 0.8476779360850842, 0.8607420270039438, 0.8732624548099196, 0.8852313113324539, 0.8966410367852339, 0.9074844245411204, 0.9177546256839781, 0.9274451533346633, 0.9365498867481886, 0.9450630751798055, 0.952979341517219, 0.9602936856769427, 0.9670014877624343, 0.9730985109821256, 0.9785809043254708, 0.983445204995331, 0.9876883405951363, 0.991307631069507, 0.9943007903969976, 0.99666592803403, 0.998401550108975, 0.9995065603657315, 0.9999802608561371, 0.9998223523808091, 0.999032934678125, 0.9976125063612249, 0.995561964603081, 0.9928826045698134, 0.9895761186026508, 0.9856445951489982, 0.9810905174433345, 0.9759167619387483, 0.9701265964901072, 0.9637236782900078, 0.956712051558833, 0.9490961449902934, 0.9408807689542295, 0.9320711124582106, 0.9226727398701151, 0.9126915874035038, 0.9021339593682045, 0.8910065241883703, 0.8793163101905596, 0.8670707011644873, 0.8542774316993005, 0.8409445822981677, 0.8270805742745693, 0.8126941644330943, 0.7977944395385723, 0.7823908105765904, 0.7664930068093533, 0.750111069630464, 0.7332553462225657, 0.7159364830218282, 0.698165418993481, 0.6799533787224183, 0.6613118653236523, 0.642252653176586, 0.6227877804881153, 0.6029295416890288, 0.5826904796685816, 0.5620833778521257, 0.5411212521268841, 0.5198173426207071, 0.4981851053395021, 0.4762382036679394, 0.45399049973954847, 0.43145604568096213, 0.40864907473635365, 0.38558399227740264, 0.3622753667045533, 0.33873792024528715, 0.31498651965531554, 0.29103616682827055, 0.2669019893203758, 0.24259923079540915, 0.2181432413965458, 0.19354946805086506, 0.16883344471274025, 0.1440107825522601, 0.11909716009486515, 0.09410831331851129, 0.06906002571440432, 0.043968118317864985, 0.01884843971540982, -0.006283143965555744, -0.031410759078123525, -0.0565185344820182, -0.08159061156816384, -0.10661115427526463, -0.13156435909228567, -0.15643446504023248, -0.18120576362713742, -0.20586260876987986, -0.2303894266765876, -0.25477072568337766, -0.27899110603923694, -0.30303526963276656, -0.32688802965494707, -0.3505343201912621, -0.37395920573780206, -0.3971478906347808, -0.420085728411805, -0.4427582310388989, -0.4651510780774669, -0.487250125725327, -0.509041415750377, -0.5305111843067263, -0.5516458706284331, -0.5724321255945924, -0.5928568201610595, -0.6129070536529755, -0.6325701619131333, -0.6518337253008755, -0.6706855765367262, -0.689113808387343, -0.7071067811865511, -0.7246531301870491, -0.7417417727387405, -0.7583619152887221, -0.7745030601987332, -0.7901550123756887, -0.8053078857111279, -0.819952109325449, -0.8340784336131749, -0.8476779360850785, -0.8607420270039455, -0.8732624548099213, -0.8852313113324555, -0.8966410367852354, -0.9074844245411159, -0.9177546256839795, -0.9274451533346645, -0.9365498867481898, -0.9450630751798066, -0.9529793415172156, -0.9602936856769437, -0.9670014877624352, -0.9730985109821264, -0.9785809043254716, -0.9834452049953315, -0.9876883405951369, -0.9913076310695075, -0.9943007903969979, -0.9966659280340302, -0.9984015501089751, -0.9995065603657316, -0.9999802608561371, -0.9998223523808091, -0.9990329346781249, -0.9976125063612246, -0.9955619646030807, -0.992882604569813, -0.9895761186026524, -0.9856445951489976, -0.9810905174433339, -0.9759167619387475, -0.9701265964901064, -0.9637236782900107, -0.956712051558832, -0.9490961449902923, -0.9408807689542283, -0.9320711124582094, -0.9226727398701193, -0.9126915874035023, -0.9021339593682031, -0.8910065241883688, -0.879316310190558, -0.8670707011644926, -0.8542774316992987, -0.8409445822981658, -0.8270805742745674, -0.8126941644330923, -0.7977944395385702, -0.7823908105765883, -0.7664930068093511, -0.7501110696304618, -0.7332553462225634, -0.7159364830218258, -0.6981654189934785, -0.6799533787224159, -0.6613118653236603, -0.6422526531765833, -0.6227877804881127, -0.6029295416890261, -0.5826904796685788, -0.5620833778521346, -0.5411212521268812, -0.5198173426207042, -0.4981851053394991, -0.4762382036679364, -0.4539904997395581, -0.431456045680959, -0.40864907473635054, -0.3855839922773995, -0.36227536670455013, -0.3387379202452973, -0.31498651965531227, -0.2910361668282673, -0.26690198932038617, -0.24259923079540582, -0.21814324139654245, -0.1935494680508617, -0.16883344471273687, -0.14401078255225672, -0.11909716009487586, -0.09410831331850787, -0.06906002571441508, -0.04396811831786156, -0.0188484397154206, 0.006283143965559174, 0.03141075907812695, 0.056518534482021626, 0.0815906115681531, 0.10661115427525392, 0.13156435909227499, 0.15643446504023586, 0.18120576362712681, 0.20586260876988322, 0.2303894266765771, 0.254770725683381, 0.2789911060392266, 0.30303526963276983, 0.3268880296549369, 0.350534320191252, 0.37395920573779207, 0.39714789063478395, 0.4200857284117952, 0.44275823103890194, 0.46515107807745737, 0.48725012572533, 0.5090414157503677, 0.5305111843067292, 0.5516458706284241, 0.5724321255945952, 0.5928568201610622, 0.6129070536529783, 0.632570161913125, 0.651833725300878, 0.6706855765367181, 0.6891138083873455, 0.7071067811865436, 0.7246531301870417, 0.7417417727387429, 0.7583619152887244, 0.7745030601987353, 0.7901550123756909, 0.8053078857111214, 0.8199521093254509, 0.834078433613169, 0.8476779360850804, 0.8607420270039473, 0.8732624548099159, 0.885231311332457, 0.896641036785237, 0.9074844245411173, 0.9177546256839809, 0.9274451533346605, 0.9365498867481911, 0.9450630751798077, 0.9529793415172167, 0.9602936856769446, 0.9670014877624361, 0.9730985109821272, 0.9785809043254723, 0.9834452049953296, 0.9876883405951374, 0.9913076310695079, 0.9943007903969984, 0.9966659280340305, 0.9984015501089746, 0.9995065603657317, 0.9999802608561371, 0.999822352380809, 0.9990329346781247, 0.9976125063612253, 0.9955619646030803, 0.9928826045698126, 0.9895761186026519, 0.985644595148997, 0.981090517443336, 0.9759167619387468, 0.9701265964901056, 0.9637236782900098, 0.956712051558831, 0.9490961449902912, 0.9408807689542271, 0.9320711124582082, 0.922672739870118, 0.912691587403501, 0.9021339593682015, 0.8910065241883672, 0.8793163101905563, 0.8670707011644909, 0.8542774316992969, 0.840944582298164, 0.8270805742745654, 0.8126941644330903, 0.7977944395385768, 0.7823908105765862, 0.7664930068093488, 0.7501110696304595, 0.733255346222561, 0.7159364830218333, 0.6981654189934761, 0.6799533787224133, 0.6613118653236577, 0.6422526531765806, 0.6227877804881211, 0.6029295416890234, 0.5826904796685759, 0.5620833778521318, 0.5411212521268783, 0.5198173426207133, 0.49818510533949617, 0.4762382036679334, 0.453990499739555, 0.4314560456809559, 0.4086490747363474, 0.3855839922773963, 0.3622753667045469, 0.3387379202452941, 0.314986519655309, 0.291036166828264, 0.26690198932038284, 0.2425992307954025, 0.21814324139655297, 0.19354946805085835, 0.16883344471273348, 0.14401078255225333, 0.11909716009487245, 0.0941083133185186, 0.06906002571441165, 0.04396811831785813, 0.018848439715417168, -0.0062831439655626035, -0.03141075907811618, -0.05651853448202505, -0.08159061156815652, -0.10661115427525733, -0.13156435909227837, -0.1564344650402252, -0.18120576362713017, -0.20586260876988655, -0.23038942667658044, -0.2547707256833843, -0.2789911060392299, -0.3030352696327731, -0.3268880296549401, -0.35053432019125524, -0.37395920573779523, -0.39714789063478706, -0.4200857284117983, -0.44275823103890505, -0.4651510780774479, -0.487250125725333, -0.5090414157503707, -0.530511184306732, -0.551645870628427, -0.5724321255945864, -0.5928568201610536, -0.6129070536529809, -0.6325701619131165, -0.6518337253008807, -0.6706855765367101, -0.689113808387348, -0.707106781186546, -0.724653130187044, -0.7417417727387356, -0.7583619152887173, -0.7745030601987285, -0.790155012375693, -0.8053078857111151, -0.8199521093254529, -0.8340784336131709, -0.8476779360850821, -0.8607420270039418, -0.8732624548099176, -0.885231311332452, -0.8966410367852384, -0.9074844245411128, -0.9177546256839823, -0.9274451533346617, -0.9365498867481922, -0.9450630751798043, -0.9529793415172177, -0.9602936856769416, -0.9670014877624333, -0.9730985109821246, -0.9785809043254731, -0.9834452049953302, -0.9876883405951379, -0.9913076310695066, -0.9943007903969987, -0.9966659280340296, -0.9984015501089748, -0.9995065603657314, -0.9999802608561371, -0.999822352380809, -0.9990329346781246, -0.9976125063612251, -0.99556196460308, -0.9928826045698138, -0.9895761186026515, -0.9856445951489988, -0.9810905174433353, -0.975916761938746, -0.9701265964901047, -0.9637236782900088, -0.95671205155883, -0.9490961449902946, -0.940880768954226, -0.9320711124582121, -0.9226727398701167, -0.9126915874034995, -0.9021339593682062, -0.8910065241883657, -0.8793163101905547, -0.8670707011644893, -0.854277431699295, -0.8409445822981698, -0.8270805742745635, -0.8126941644330883, -0.7977944395385747, -0.782390810576584, -0.7664930068093557, -0.7501110696304573, -0.7332553462225587, -0.715936483021831, -0.6981654189934736, -0.6799533787224108, -0.6613118653236552, -0.6422526531765781, -0.6227877804881184, -0.6029295416890206, -0.5826904796685731, -0.5620833778521289, -0.5411212521268755, -0.5198173426207104, -0.4981851053394932, -0.47623820366793035, -0.45399049973955197, -0.4314560456809528, -0.4086490747363572, -0.38558399227739315, -0.3622753667045437, -0.33873792024529087, -0.3149865196553058, -0.2910361668282743, -0.26690198932037956, -0.24259923079539916, -0.21814324139654964, -0.193549468050855, -0.1688334447127441, -0.14401078255224992, -0.11909716009486905, -0.09410831331851519, -0.06906002571440822, -0.0439681183178547, -0.01884843971541374, 0.006283143965566034, 0.031410759078119604, 0.056518534482028475, 0.08159061156815993, 0.10661115427526073, 0.13156435909228179, 0.1564344650402286, 0.18120576362713356, 0.2058626087698899, 0.23038942667658377, 0.25477072568338766, 0.2789911060392195, 0.3030352696327764, 0.3268880296549434, 0.35053432019125846, 0.37395920573779845, 0.3971478906347772, 0.4200857284118015, 0.4427582310389081, 0.4651510780774509, 0.487250125725336, 0.5090414157503613, 0.5305111843067349, 0.5516458706284298, 0.5724321255945892, 0.5928568201610563, 0.6129070536529724, 0.6325701619131192, 0.6518337253008832, 0.6706855765367127, 0.6891138083873505, 0.7071067811865483, 0.7246531301870464, 0.741741772738738, 0.7583619152887195, 0.7745030601987306, 0.7901550123756951, 0.8053078857111171, 0.8199521093254549, 0.8340784336131649, 0.8476779360850839, 0.8607420270039435, 0.8732624548099193, 0.8852313113324537, 0.8966410367852337, 0.9074844245411142, 0.9177546256839836, 0.9274451533346577, 0.9365498867481934, 0.9450630751798007, 0.9529793415172187, 0.9602936856769426, 0.9670014877624342, 0.9730985109821255, 0.9785809043254708, 0.9834452049953283, 0.9876883405951384, 0.9913076310695051, 0.994300790396999, 0.9966659280340299, 0.9984015501089749, 0.9995065603657315, 0.9999802608561371, 0.9998223523808091, 0.9990329346781245, 0.9976125063612259, 0.9955619646030797, 0.9928826045698151, 0.9895761186026509, 0.9856445951489983, 0.9810905174433346, 0.9759167619387484, 0.9701265964901074, 0.9637236782900117, 0.956712051558829, 0.9490961449902979, 0.9408807689542248, 0.9320711124582108, 0.9226727398701153, 0.912691587403504, 0.9021339593682047, 0.8910065241883706, 0.8793163101905598, 0.8670707011644946, 0.8542774316992933, 0.840944582298168, 0.8270805742745616, 0.8126941644330946, 0.7977944395385727, 0.7823908105765908, 0.7664930068093536, 0.7501110696304644, 0.7332553462225564, 0.7159364830218286, 0.6981654189934712, 0.6799533787224188, 0.6613118653236526, 0.6422526531765863, 0.6227877804881157, 0.6029295416890292, 0.5826904796685819, 0.5620833778521261, 0.5411212521268726, 0.5198173426207076, 0.49818510533949023, 0.47623820366793984, 0.4539904997395489, 0.4314560456809626, 0.4086490747363541, 0.38558399227739, 0.36227536670455374, 0.33873792024528765, 0.3149865196553025, 0.291036166828271, 0.26690198932037623, 0.24259923079540963, 0.21814324139654628, 0.1935494680508516, 0.16883344471274073, 0.14401078255224653, 0.11909716009486565, 0.09410831331851177, 0.06906002571440481, 0.04396811831786547, 0.01884843971541031, -0.006283143965569464, -0.03141075907812303, -0.056518534482031896, -0.08159061156814919, -0.10661115427526414, -0.13156435909228517, -0.15643446504023198, -0.18120576362713692, -0.20586260876987936, -0.23038942667658713, -0.25477072568339093, -0.27899110603922284, -0.30303526963277966, -0.3268880296549332, -0.3505343201912617, -0.3739592057378016, -0.39714789063478034, -0.4200857284118046, -0.4427582310389112, -0.46515107807745393, -0.487250125725339, -0.5090414157503643, -0.5305111843067378, -0.5516458706284327, -0.572432125594592, -0.5928568201610591, -0.6129070536529752, -0.6325701619131219, -0.6518337253008859, -0.6706855765367152, -0.6891138083873529, -0.7071067811865408, -0.7246531301870488, -0.7417417727387402, -0.7583619152887218, -0.7745030601987328, -0.7901550123756884, -0.8053078857111191, -0.8199521093254568, -0.8340784336131668, -0.8476779360850858, -0.8607420270039381, -0.8732624548099209, -0.8852313113324553, -0.8966410367852352, -0.9074844245411157, -0.9177546256839849, -0.927445153334659, -0.9365498867481946, -0.9450630751798018, -0.9529793415172199, -0.9602936856769436, -0.9670014877624351, -0.9730985109821263, -0.9785809043254715, -0.9834452049953288, -0.987688340595139, -0.9913076310695056, -0.9943007903969995, -0.996665928034029, -0.9984015501089751, -0.9995065603657316, -0.9999802608561371, -0.9998223523808091, -0.9990329346781249, -0.9976125063612257, -0.9955619646030793, -0.9928826045698147, -0.9895761186026505, -0.985644595149, -0.981090517443334, -0.9759167619387477, -0.9701265964901065, -0.9637236782900108, -0.9567120515588322, -0.9490961449902969, -0.9408807689542237, -0.9320711124582147, -0.922672739870114, -0.9126915874035025, -0.9021339593682033, -0.891006524188369, -0.8793163101905582, -0.8670707011644928, -0.8542774316992915, -0.8409445822981738, -0.8270805742745596, -0.8126941644331008, -0.7977944395385705, -0.7823908105765887, -0.7664930068093514, -0.7501110696304621, -0.7332553462225637, -0.7159364830218361, -0.6981654189934686, -0.6799533787224267, -0.66131186532365, -0.6422526531765946, -0.622787780488113, -0.6029295416890265, -0.5826904796685791, -0.562083377852135, -0.5411212521268817, -0.5198173426207168, -0.49818510533948723, -0.47623820366794933, -0.45399049973954586, -0.43145604568095947, -0.408649074736351, -0.3855839922773999, -0.36227536670455057, -0.33873792024529775, -0.3149865196552992, -0.2910361668282813, -0.26690198932037296, -0.2425992307954063, -0.21814324139654295, -0.19354946805086218, -0.16883344471273734, -0.14401078255225722, -0.11909716009487635, -0.0941083133185225, -0.06906002571440138, -0.04396811831786204, -0.01884843971540688, 0.006283143965558684, 0.03141075907812646, 0.056518534482021134, 0.08159061156815262, 0.10661115427525343, 0.13156435909227449, 0.15643446504023537, 0.1812057636271403, 0.20586260876988272, 0.23038942667659046, 0.25477072568338055, 0.2789911060392261, 0.3030352696327694, 0.32688802965493646, 0.35053432019126485, 0.3739592057378048, 0.3971478906347835, 0.4200857284118077, 0.44275823103890155, 0.465151078077457, 0.48725012572532955, 0.5090414157503672, 0.5305111843067408, 0.5516458706284237, 0.5724321255945949, 0.5928568201610619, 0.6129070536529778, 0.6325701619131245, 0.6518337253008777, 0.6706855765367178, 0.6891138083873555, 0.7071067811865432, 0.0, 0.0, 0.0, 0.0, 0.0, 0.0, 0.0, 0.0, 0.0, 0.0, 0.0, 0.0, 0.0, 0.0, 0.0, 0.0, 0.0, 0.0, 0.0]
  in  "Send waveform to AWG":bool
  out "Ring Text.Text":string
  out "Ring 2":u16(ring)
  in  "Ring":u16(ring)
  out "Waveform name indicator":u16
  in  "stop":bool
  out "appended path 2":path=path "D:/Heidelberg/Setup/Microwave/Tabor/Tabor_SE5082/waveform_preset/timing_v63-cwBlue_preset03.dat"
  in  "Save as Preset #":u16(ring)=3 items=["0", "1", "2", "3", "4", "5", "6", "7", "8", "9", "10", "11", "12", "13", "14", "15", "16", "17", "18", "19", "20", "21", "22", "23", "24", "25"]
  in  "name or relative path":string
  out "appended path":path
  out "Parent Directory (+ Relative)":path=path "D:/Heidelberg/Setup/Microwave/Tabor/Tabor_SE5082"
  out "path":path=path "D:/Heidelberg/Setup/Microwave/Tabor/Tabor_SE5082/test_GUI_with_seq.vi"
  in  "AWG sequence_variables":T3={"Sampling rate"=5000000000, "Channel"=1, "Sequence name"=0, "Save sequence"=FALSE, "Load waveform"=TRUE, "Waveform"=[{"Sequence on"=TRUE, "segment name"=0, "repeat"="1", "delay time"="0"}, {"Sequence on"=TRUE, "segment name"=1, "repeat"="1", "delay time"="1"}, {"Sequence on"=TRUE, "segment name"=2, "repeat"="1", "delay time"="0.5"}]} {"Sequence name" items=["Init X", "WAHUHA", "Readout X", "New waveform..."]; "Channel" format="%.0p"; "Sampling rate" format="%.0p"; "Waveform"."segment name" items=["Init X", "WAHUHA", "Readout X"]}
  # "Note: if use high freq > 20 MHz: the tiepie scope cannot capture the pulse and cause the amplitude glitch."
  # "No."
  # "freq (MHz)"
  # "phase  (deg)"
  # "amplitude (0-1)"
  # "duration (us)"
  # "envelope"
  # "No."
  # "freq (MHz)"
  # "phase  (deg)"
  # "amplitude (0-1)"
  # "duration (us)"
  # "envelope"
  # "Max 5 GSa/s"
  # "1 or 2"
  # "ON?"
  # "segment name"
  # "repeat"
  # "delay time (us)"
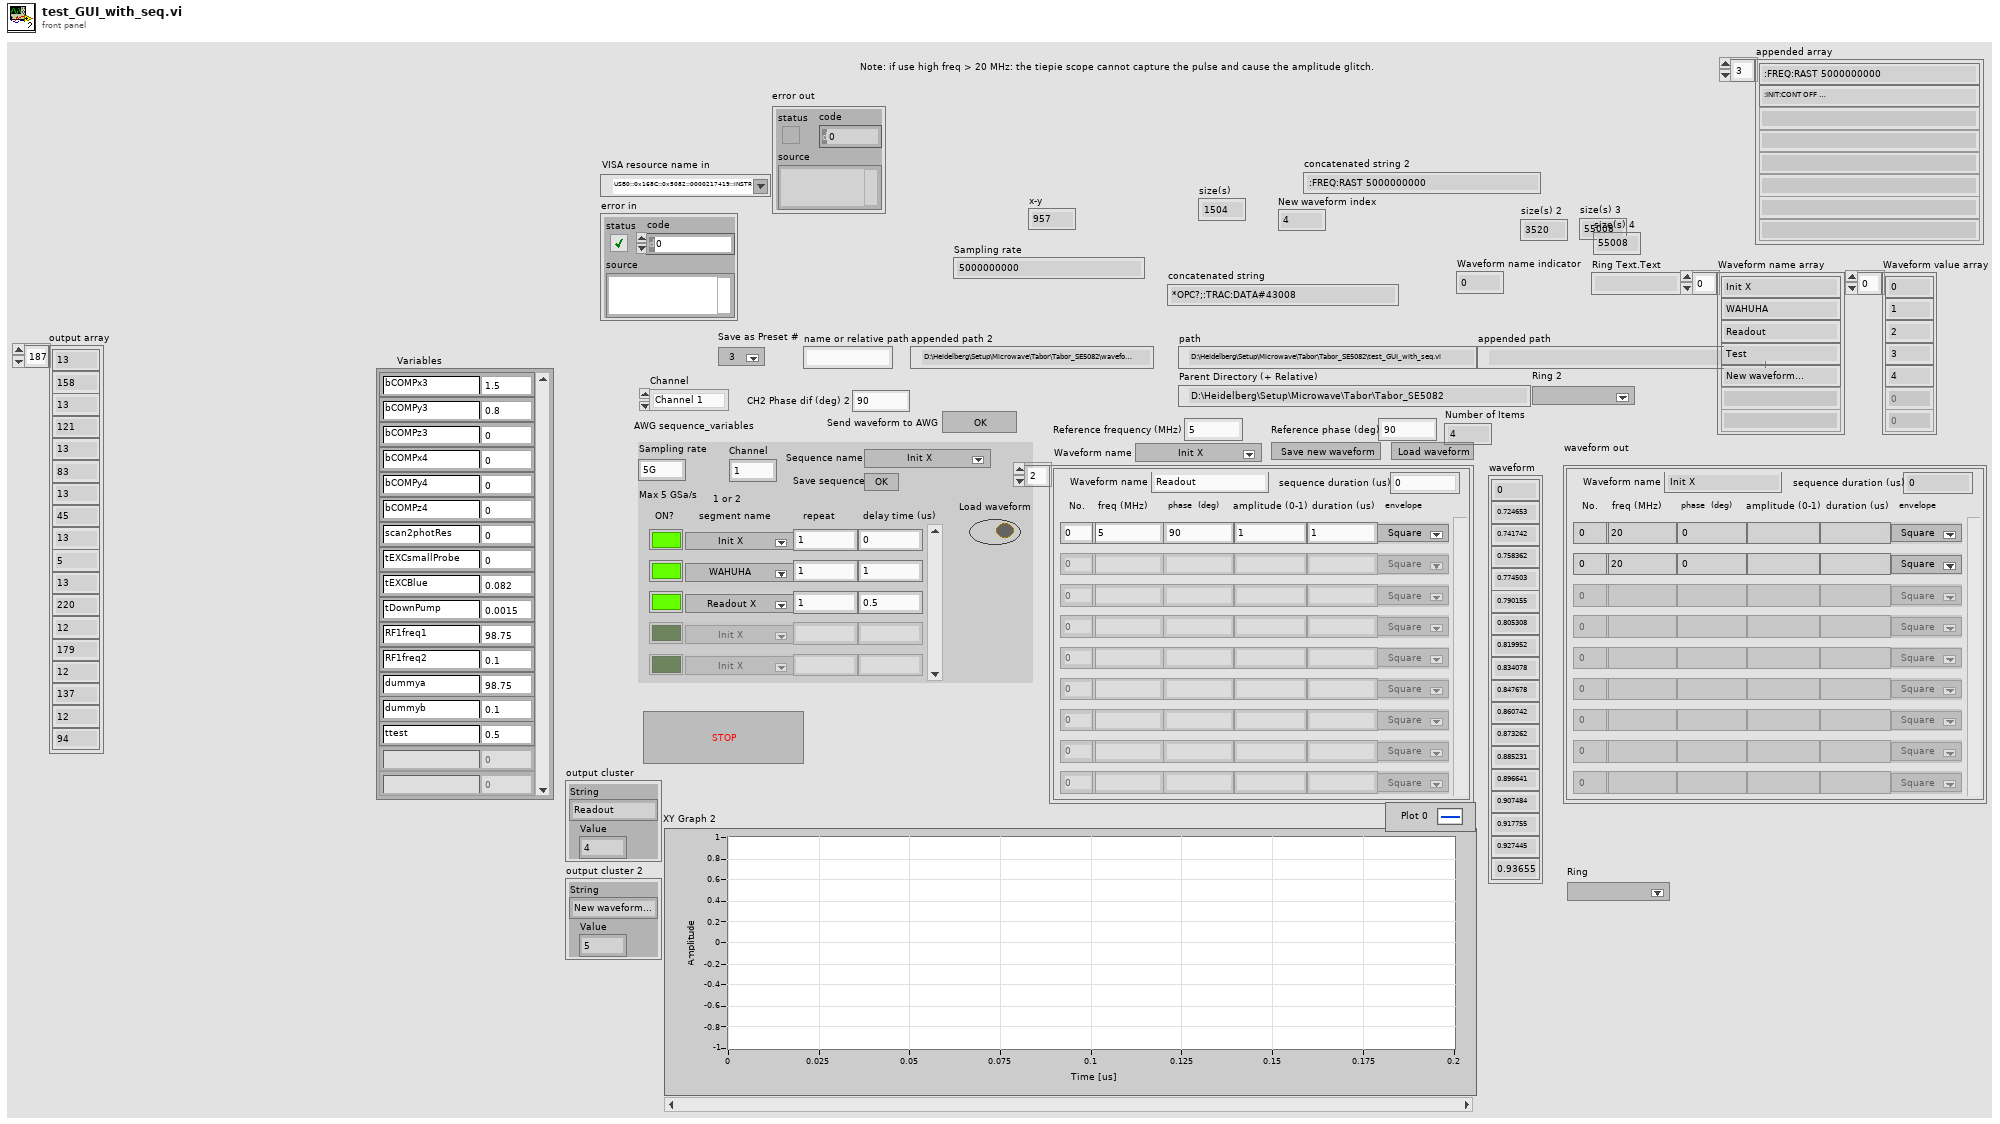
[diagram p1: front panel]
types:
  T1 = typedef "waveform_variables_new.ctl" = cluster{"Waveform name":string, "sequence duration (us)":dbl, "Waveform":cluster{"Segment number":i32, "frequency":string, "phase":string, "amplitude":string, "duration":string, "envelope":u16}[]}[]
  T2 = typedef "variables.ctl" = cluster{"Value":dbl, "Variable":string, "Save with Image":bool}[]
  T3 = typedef "sequence_variables.ctl" = cluster{"Sampling rate":i64, "Channel":i8, "Sequence name":u16, "Save sequence":bool, "Load waveform":bool, "Waveform":cluster{"Sequence on":bool, "segment name":u16, "repeat":string, "delay time":string}[]}
  T4 = cluster{"Waveform name":string, "sequence duration (us)":dbl, "Waveform":cluster{"Segment number":i32, "frequency":string, "phase":string, "amplitude":string, "duration":string, "envelope":u16}[]}
  T5 = cluster{"Waveform name":string, "sequence duration (us)":dbl, "Waveform":cluster{"Segment number":i32, "frequency":string, "phase":string, "amplitude":string, "duration":string, "envelope":u16}[]}[]
  T6 = typedef "LVStringsAndValuesArrayTypeDef_U16.ctl" = cluster{"String":string, "Value":u16}[]
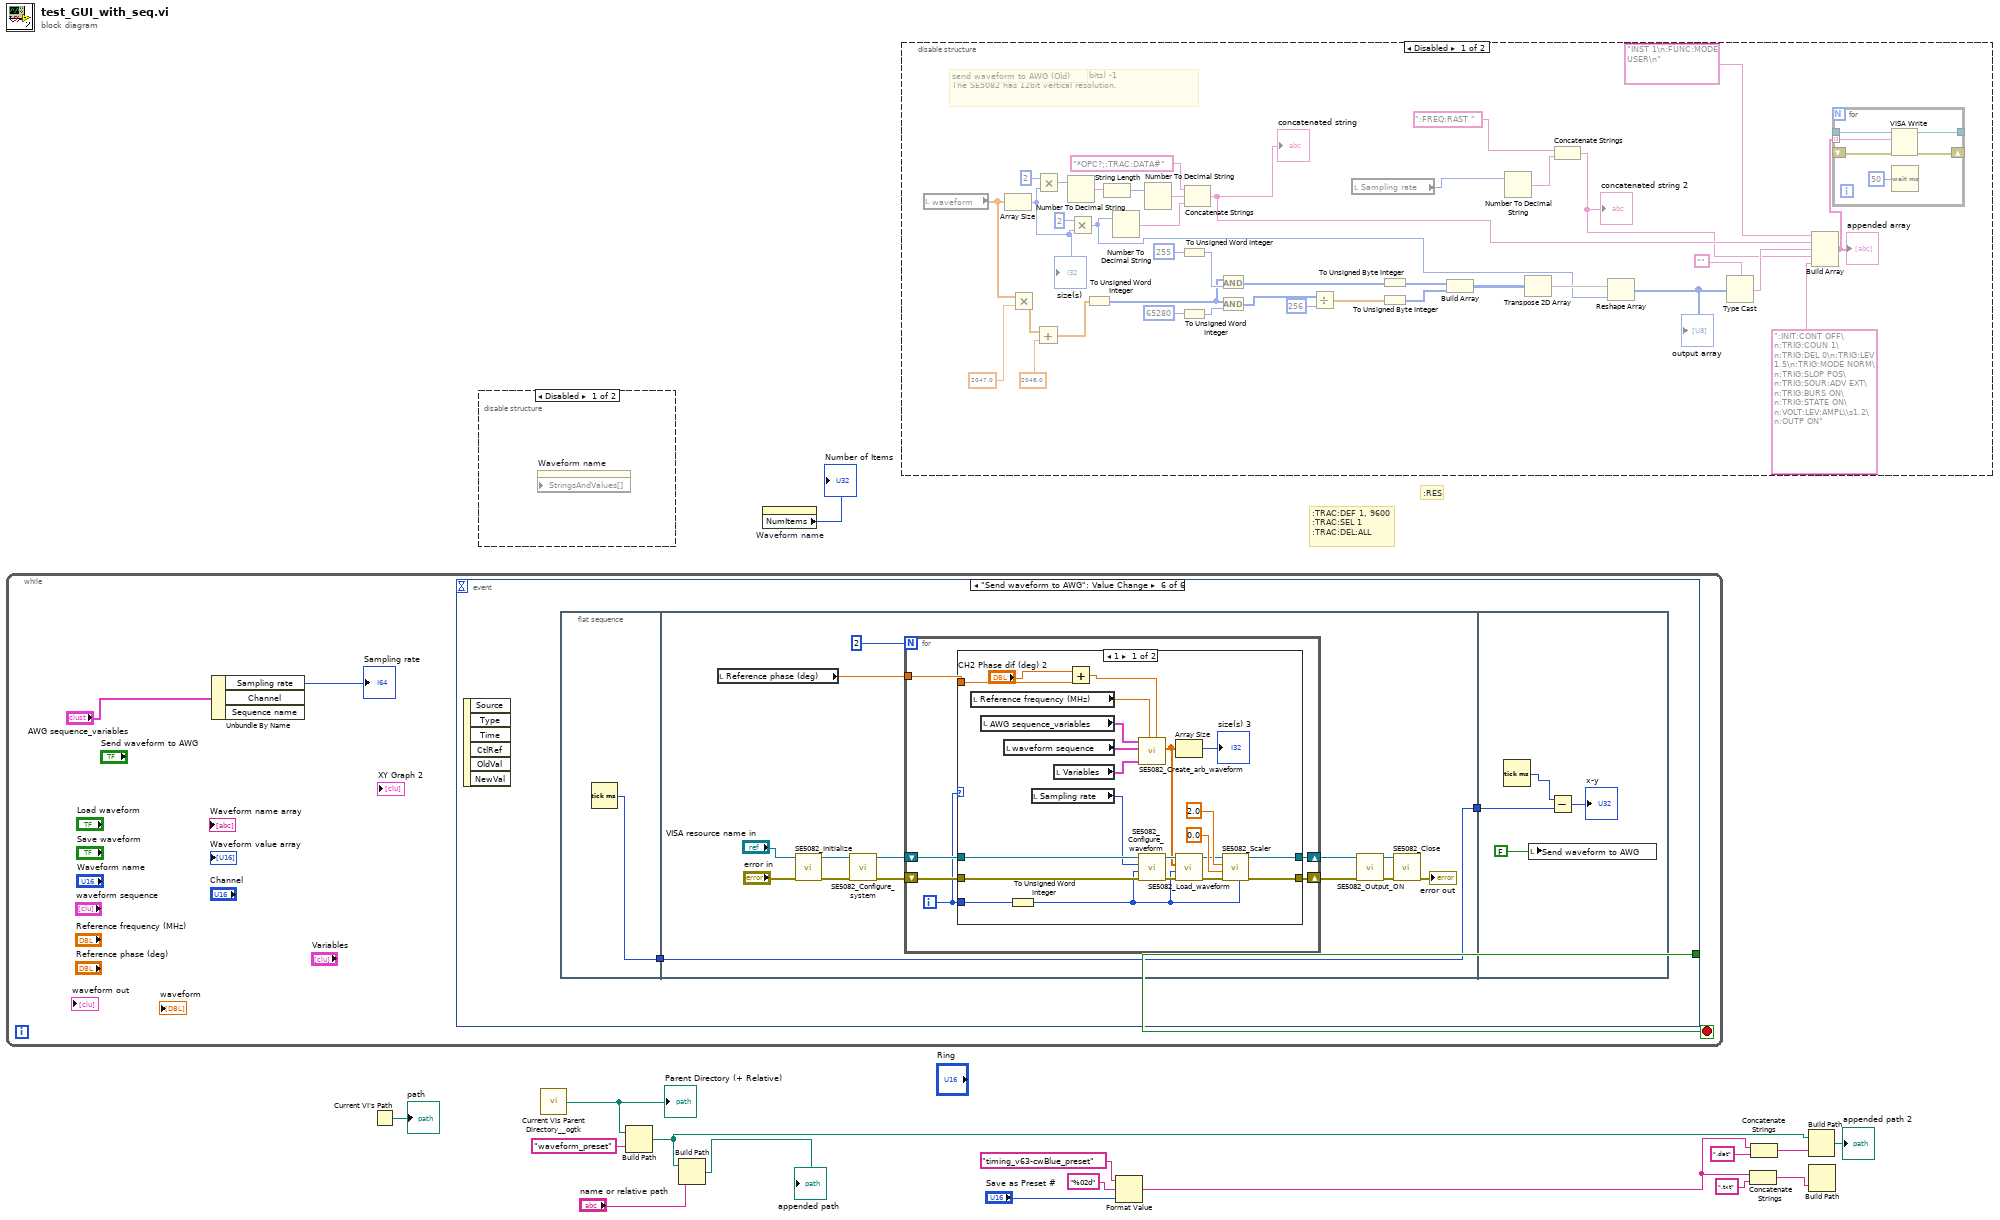
[diagram p0: block diagram]
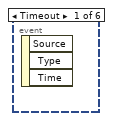
[diagram p4: hidden frame]
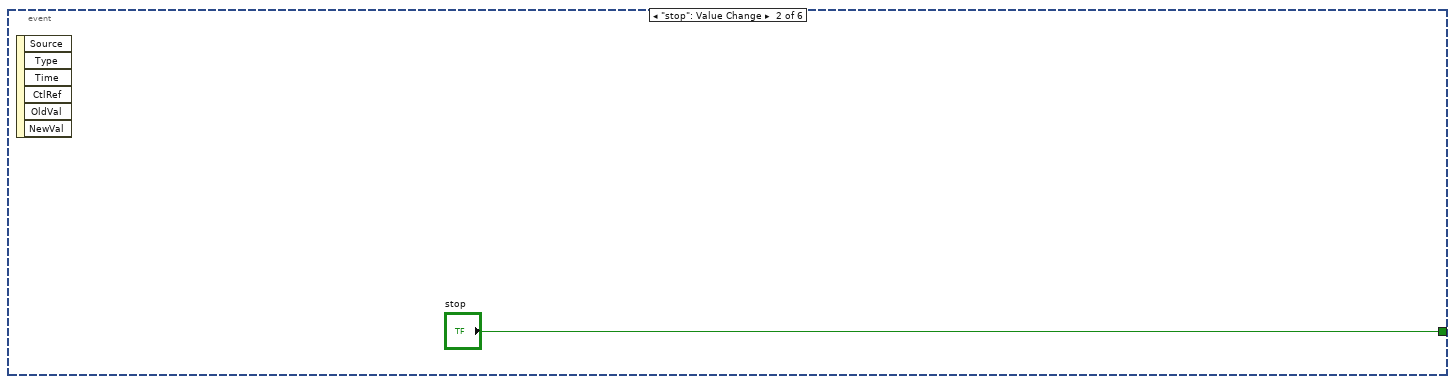
[diagram p5: hidden frame]
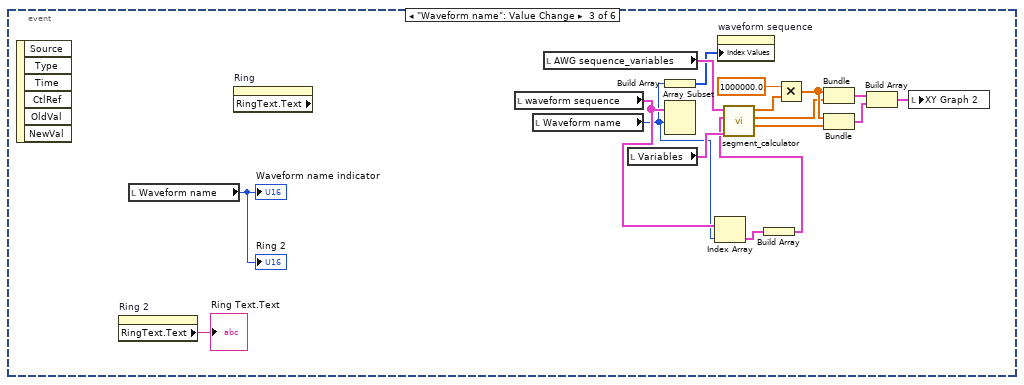
[diagram p6: hidden frame]
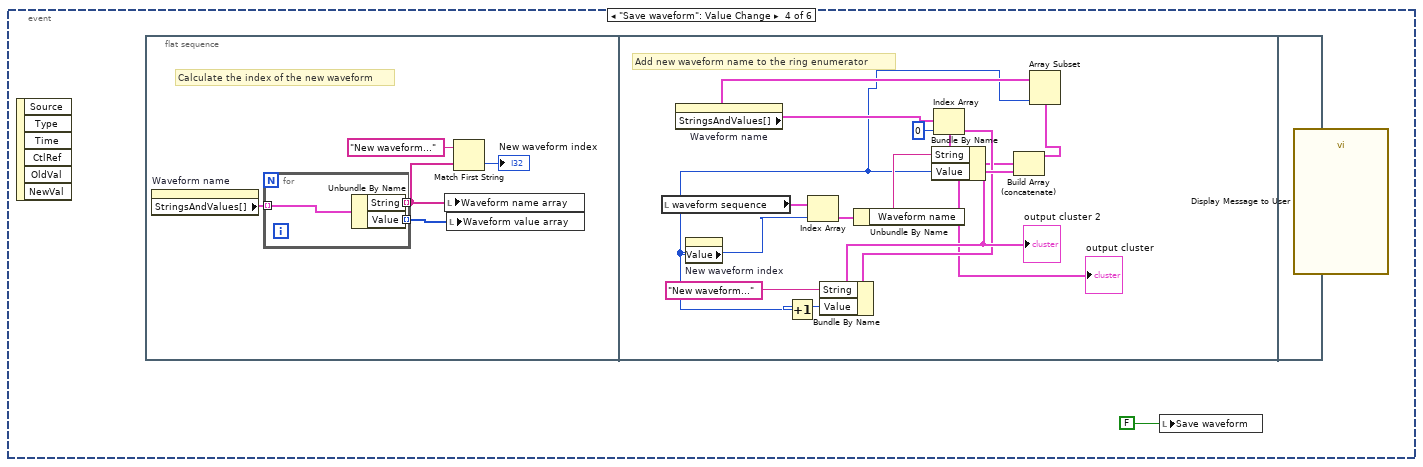
[diagram p7: hidden frame]
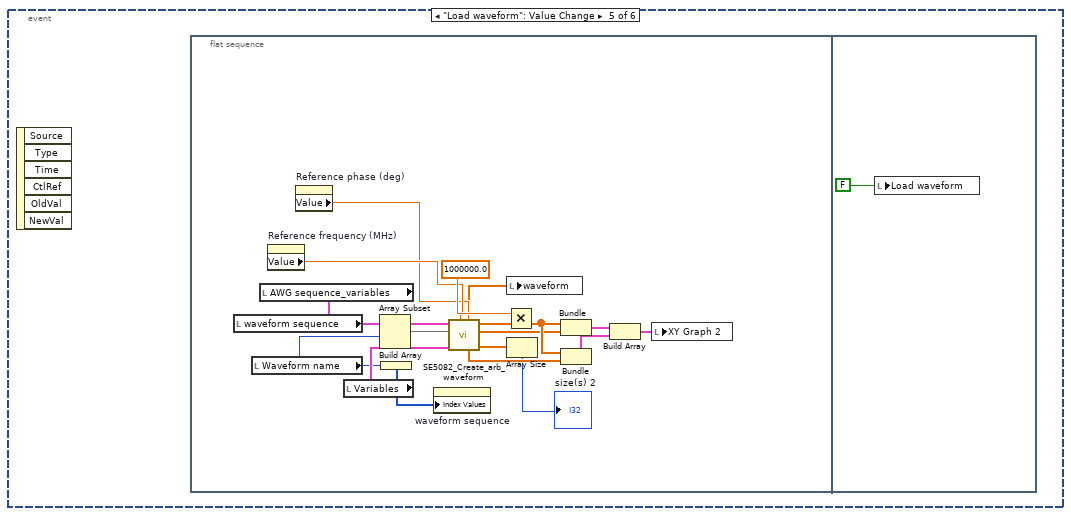
[diagram p8: hidden frame]
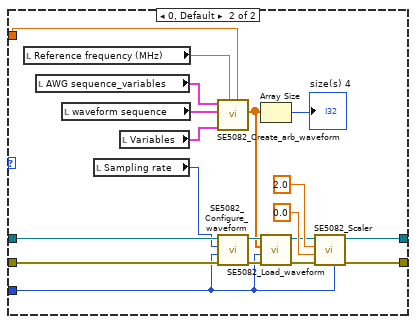
[diagram p9: hidden frame]
diagram:
  # ":RES"
  # ":TRAC:DEF 1, 9600\n:TRAC:SEL 1\n:TRAC:DEL:ALL"
  n1 = while {
    stop <- w19 stop-if-true
    n2 = Unbundle By Name("AWG sequence_variables") -> ("Sampling rate"=→"Sampling rate":i64)  [unwired: 2 out]
    n3 = event shown="[5] \"Send waveform to AWG\": Value Change" {
      selector: _ -> [_ _ _ _ _ _]
      dyn-events: _ -> [_ _ _ _ _ _]
      timeout: _ -> [_ _ _ _ _ _]
      tunnel: [_ "stop" _ _ _ _] -> w19
      event Timeout {
        n4 = event-data() -> ()  [unwired: 1 in, 3 out]
      }
      event "stop": Value Change {
        n5 = event-data() -> ()  [unwired: 1 in, 6 out]
      }
      event "Waveform name": Value Change {
        n6 = event-data() -> ()  [unwired: 1 in, 6 out]
        n7 = property on="Ring 2" class="Ring (strict)"() -> ("RingText.Text"=→"Ring Text.Text":string)  [unwired: 2 in, 2 out]
        n8 = local read "Waveform name"() -> (→"Waveform name indicator" →"Ring 2":u16)
        n9 = property on="Ring" class="Ring (strict)" props=["RingText", "Text"]() -> ()  [unwired: 2 in, 3 out]
        n10 = local read "waveform sequence"() -> (w23:T1)
        n11 = local read "Waveform name"() -> (w22:u16)
        n12 = local read "AWG sequence_variables"() -> (w28:T3)
        n13 = local read "Variables"() -> (w35:T2)
        n14 = Build Array(w22) -> (w27:u16[])
        n15 = Array Subset(array=w23, index=w22) -> ()  [unwired: 1 in, 1 out]
        n16 = Index Array(array=w23, index=w22) -> (element=w24:T4)
        n17 = property on="waveform sequence" class="Arr (strict)"("Index Values"=w27) -> ()  [unwired: 2 in, 2 out]
        n18 = Build Array(w24) -> (w21:T5)
        n19 = call "segment_calculator.vi"("Variables"=w35, "waveform sequence"=w21, "AWG sequence_variables"=w28) -> ("ref"=w33:dbl[], "y"=w30:dbl[], "x"=w29:dbl[])  [unwired: 5 in]
        n20 = Multiply(x=1000000.0, y=w29) -> (x*y=w32:dbl[])
        n21 = Bundle(w32, "y"=w30) -> (w31:cluster{dbl[], "y":dbl[]})  [unwired: 1 in]
        n22 = Bundle(w32, "ref"=w33) -> (w34:cluster{dbl[], "ref":dbl[]})  [unwired: 1 in]
        n23 = Build Array(w31, w34) -> (w26:cluster{dbl[], "ref":dbl[]}[])
        n24 = local write "XY Graph 2"(w26) -> ()
      }
      event "Save waveform": Value Change {
        n25 = event-data() -> ()  [unwired: 1 in, 6 out]
        n26 = flat-sequence {
          frame #0 {
            # "Calculate the index of the new waveform"
            n27 = property on="Waveform name" class="Ring (strict)"() -> ("StringsAndValues[]"=w43:T6)  [unwired: 2 in, 2 out]
            n28 = for {
              tunnel: w43 -> [w46] mode=indexing
              tunnel: [w45] -> w40 mode=indexing
              tunnel: [w44] -> w39 mode=indexing
              n29 = Unbundle By Name(w46) -> ("String"=w45:string, "Value"=w44:u16)
            }
            n30 = local write "Waveform name array"(w40) -> ()
            n31 = local write "Waveform value array"(w39) -> ()
            n32 = Match First String(2:w40, 3:"New waveform..." ("string")) -> (0:→"New waveform index":i32)  [unwired: 1 out]
          }
          frame #1 {
            # "Add new waveform name to the ring enumerator"
            n33 = local read "waveform sequence"() -> (w52:T1)
            n34 = property on="Waveform name" class="Ring (strict)"() -> ("StringsAndValues[]"=w49:T6)  [unwired: 2 in, 2 out]
            n35 = property on="New waveform index" class="DigNum (strict)"() -> ("Value"=w47:i32)  [unwired: 2 in, 2 out]
            n36 = Increment(x=w47) -> (x+1=w58:i32)
            n37 = Index Array(array=w52, index=w47) -> (element=w51:T4)
            n38 = Unbundle By Name(w51) -> ("Waveform name"=w50:string)
            n39 = Index Array(array=w49, index=0) -> (element=w56:cluster{"String":string, "Value":u16})
            n40 = Bundle By Name(cluster=w56, "String"="New waveform..." ("string"), "Value"=w58) -> (w57:cluster{"String":string, "Value":u16})
            "output cluster 2" <- w57
            n41 = Bundle By Name(cluster=w56, "String"=w50, "Value"=w47) -> (w55:cluster{"String":string, "Value":u16})
            "output cluster" <- w55
            n42 = Array Subset(array=w49, length=w47) -> (w48:T6)  [unwired: 1 in]
            n43 = Build Array (concatenate)(w48, w55, w57) -> ()  [unwired: 1 out]
          }
          frame #2 {
          }
        }
        n44 = local write "Save waveform"(FALSE ("Save waveform")) -> ()
        n45 = call "Display Message to User"() -> ()  [unwired: 10 in, 2 out]
      }
      event "Load waveform": Value Change {
        n46 = event-data() -> ()  [unwired: 1 in, 6 out]
        n47 = flat-sequence {
          frame #0 {
            n48 = local read "waveform sequence"() -> (w67:T1)
            n49 = local read "Waveform name"() -> (w65:u16)
            n50 = local read "AWG sequence_variables"() -> (w68:T3)
            n51 = property on="Reference frequency (MHz)" class="DigNum (strict)"() -> ("Value"=w61:dbl)  [unwired: 2 in, 2 out]
            n52 = property on="Reference phase (deg)" class="DigNum (strict)"() -> ("Value"=w60:dbl)  [unwired: 2 in, 2 out]
            n53 = local read "Variables"() -> (w75:T2)
            n54 = Array Subset(array=w67, index=w65) -> (w66:T1)  [unwired: 1 in]
            n55 = Build Array(w65) -> (w64:u16[])
            n56 = property on="waveform sequence" class="Arr (strict)"("Index Values"=w64) -> ()  [unwired: 2 in, 2 out]
            n57 = call "SE5082_Create_arb_waveform.vi"("Reference phase (deg)"=w60, "Reference frequency (MHz)"=w61, "Variables"=w75, "waveform sequence"=w66, "AWG sequence_variables"=w68) -> ("ref amplitude"=w73:dbl[], "y"=w59:dbl[], "x"=w70:dbl[])  [unwired: 4 in]
            n58 = Multiply(x=1000000.0, y=w70) -> (x*y=w72:dbl[])
            n59 = local write "waveform"(w59) -> ()
            n60 = Array Size(array=w59) -> (size(s)=→"size(s) 2":i32)
            n61 = Bundle(w72, "y"=w59) -> (w71:cluster{dbl[], "y":dbl[]})  [unwired: 1 in]
            n62 = Bundle(w72, "ref amplitude"=w73) -> (w74:cluster{dbl[], "ref amplitude":dbl[]})  [unwired: 1 in]
            n63 = Build Array(w71, w74) -> (w63:cluster{dbl[], "ref amplitude":dbl[]}[])
            n64 = local write "XY Graph 2"(w63) -> ()
          }
          frame #1 {
            n65 = local write "Load waveform"(FALSE ("Save waveform")) -> ()
          }
        }
      }
      event "Send waveform to AWG": Value Change {
        n66 = event-data() -> ()  [unwired: 1 in, 6 out]
        n67 = flat-sequence {
          tunnel: [w79] -> w78
          tunnel: w78 -> [w80]
          tunnel: [w80] -> w77
          tunnel: w77 -> [w142]
          frame #0 {
            n68 = Tick Count (ms)() -> (millisecond timer value=w79:u32)
          }
          frame #1 {
            n69 = local read "Reference phase (deg)"() -> (w93:dbl)
            n70 = call "SE5082_Initialize.vi"("error in (no error)"="error in", "VISA resource name"="VISA resource name in") -> ("error out"=w86:errorcluster, "VISA resource name out"=w87:refnum<visa-resource-name>)  [unwired: 8 in]
            n71 = call "SE5082_Configure_system.vi"("error in"=w86, "VISA resource name in"=w87) -> ("error out"=w84:errorcluster, "VISA resource name out"=w85:refnum<visa-resource-name>)  [unwired: 8 in]
            n72 = for {
              N: 2 -> [_]
              tunnel: w93 -> [w99]
              shift-right: [w96] -> w90
              shift-left: w85 -> [w98]
              shift-right: [w95] -> w89
              shift-left: w84 -> [w97]
              i -> [w94]
              n73 = case shown="1" w94 {
                tunnel: w94 -> [w100 w122]
                tunnel: w99 -> [w104 w136]
                tunnel: w98 -> [w116 w134]
                tunnel: w97 -> [w115 w133]
                tunnel: [w111 w129] -> w96
                tunnel: [w110 w128] -> w95
                frame 1 {
                  n74 = local read "Reference frequency (MHz)"() -> (w118:dbl)
                  n75 = local read "AWG sequence_variables"() -> (w121:T3)
                  n76 = local read "waveform sequence"() -> (w120:T1)
                  n77 = To Unsigned Word Integer(number=w100) -> (unsigned 16bit integer=w101:u16)
                  n78 = local read "Sampling rate"() -> (w103:i64)
                  n79 = local read "Variables"() -> (w119:T2)
                  n80 = Add(x="CH2 Phase dif (deg) 2", y=w104) -> (x+y=w105:dbl)
                  n81 = call "SE5082_Create_arb_waveform.vi"("Reference phase (deg)"=w105, "Reference frequency (MHz)"=w118, "Variables"=w119, "waveform sequence"=w120, "AWG sequence_variables"=w121) -> ("y"=w113:dbl[])  [unwired: 4 in, 2 out]
                  n82 = call "SE5082_Configure_waveform.vi"("error in"=w115, "Channel"=w101, "Sampling rate"=w103, "VISA resource name in"=w116) -> ("error out"=w114:errorcluster, "VISA resource name out"=w117:refnum<visa-resource-name>)  [unwired: 6 in]
                  n83 = Array Size(array=w113) -> (size(s)=→"size(s) 3":i32)
                  n84 = call "SE5082_Load_waveform.vi"("error in"=w114, "Channel"=w101, "waveform"=w113, "VISA resource name in"=w117) -> ("error out"=w107:errorcluster, "VISA resource name out"=w106:refnum<visa-resource-name>)  [unwired: 6 in]
                  n85 = call "SE5082_Scaler.vi"("Channel"=w101, "error in"=w107, "Voffset"=0.0, "Vpp"=2.0, "VISA resource name in"=w106) -> ("error out"=w110:errorcluster, "VISA resource name out"=w111:refnum<visa-resource-name>)  [unwired: 5 in]
                }
                frame 0, Default {
                  n86 = local read "Reference frequency (MHz)"() -> (w137:dbl)
                  n87 = local read "AWG sequence_variables"() -> (w140:T3)
                  n88 = local read "waveform sequence"() -> (w139:T1)
                  n89 = local read "Sampling rate"() -> (w123:i64)
                  n90 = local read "Variables"() -> (w138:T2)
                  n91 = call "SE5082_Create_arb_waveform.vi"("Reference phase (deg)"=w136, "Reference frequency (MHz)"=w137, "Variables"=w138, "waveform sequence"=w139, "AWG sequence_variables"=w140) -> ("y"=w131:dbl[])  [unwired: 4 in, 2 out]
                  n92 = call "SE5082_Configure_waveform.vi"("error in"=w133, "Channel"=w122, "Sampling rate"=w123, "VISA resource name in"=w134) -> ("error out"=w132:errorcluster, "VISA resource name out"=w135:refnum<visa-resource-name>)  [unwired: 6 in]
                  n93 = Array Size(array=w131) -> (size(s)=→"size(s) 4":i32)
                  n94 = call "SE5082_Load_waveform.vi"("error in"=w132, "Channel"=w122, "waveform"=w131, "VISA resource name in"=w135) -> ("error out"=w125:errorcluster, "VISA resource name out"=w124:refnum<visa-resource-name>)  [unwired: 6 in]
                  n95 = call "SE5082_Scaler.vi"("Channel"=w122, "error in"=w125, "Voffset"=0.0, "Vpp"=2.0, "VISA resource name in"=w124) -> ("error out"=w128:errorcluster, "VISA resource name out"=w129:refnum<visa-resource-name>)  [unwired: 5 in]
                }
              }
            }
            n96 = call "SE5082_Output_ON.vi"("error in"=w89, "VISA resource name in"=w90) -> ("error out"=w81:errorcluster, "VISA resource name out"=w83:refnum<visa-resource-name>)  [unwired: 8 in]
            n97 = call "SE5082_Close.vi"("error in (no error)"=w81, "VISA resource name"=w83) -> ("error out"=→"error out":errorcluster)  [unwired: 9 in]
          }
          frame #2 {
            n98 = Tick Count (ms)() -> (millisecond timer value=w143:u32)
            n99 = local write "Send waveform to AWG"(FALSE ("Send waveform")) -> ()
            n100 = Subtract(x=w143, y=w142) -> (x-y=→"x-y":u32)
          }
        }
      }
    }
  }
  n101 = Current VI's Path() -> (path=→"path":path)
  n102 = disable-structure shown="Disabled" {
    frame Disabled {
      n103 = property on="Waveform name" class="Ring (strict)" props=["StringsAndValues[]"]() -> ()  [unwired: 3 in, 2 out]
    }
    frame Enabled {
    }
  }
  n104 = call <userlib>:"Current VIs Parent Directory__ogtk.vi"() -> ("Parent Directory (+ Relative)"=w15:path)  [unwired: 5 in]
  "Parent Directory (+ Relative)" <- w15
  n105 = Build Path(base path=w15, name or relative path="waveform_preset") -> (appended path=w4:path)
  n106 = Build Path(base path=w4, name or relative path="name or relative path") -> (appended path=→"appended path":path)
  n107 = property on="Waveform name" class="Ring (strict)"() -> ("NumItems"=→"Number of Items":u32)  [unwired: 2 in, 2 out]
  n108 = disable-structure shown="Disabled" {
    frame Disabled {
      # "send waveform to AWG (Old)"
      # "vertical resolution: 2^(number of bits) -1\nThe SE5082 has 12bit vertical resolution."
      n109 = local read "waveform"() -> (w155:dbl[])
      n110 = Array Size(array=w155) -> (size(s)=w176:i32)
      "size(s)" <- w176
      n111 = Multiply(x=w155, y=2047.0) -> (x*y=w163:dbl[])
      n112 = Add(x=w163, y=2048.0) -> (x+y=w162:dbl[])
      n113 = Multiply(x=2, y=w176) -> (x*y=w183:i32)
      n114 = Number To Decimal String(number=w183) -> (decimal integer string=w180:string)  [unwired: 1 in]
      n115 = Multiply(x=2, y=w176) -> (x*y=w154:i32)
      n116 = To Unsigned Word Integer(number=w162) -> (unsigned 16bit integer=w168:u16[])
      n117 = String Length(string=w180) -> (length=w181:i32)
      n118 = Number To Decimal String(number=w154) -> (decimal integer string=w175:string)  [unwired: 1 in]
      n119 = Number To Decimal String(number=w181) -> (decimal integer string=w182:string)  [unwired: 1 in]
      n120 = To Unsigned Word Integer(number=255) -> (unsigned 16bit integer=w174:u16)
      n121 = To Unsigned Word Integer(number=65280) -> (unsigned 16bit integer=w172:u16)
      n122 = Concatenate Strings("*OPC?;:TRAC:DATA#", w182, w175) -> (w153:string)
      "concatenated string" <- w153
      n123 = And(x=w168, y=w174) -> (x .and. y?=w173:u16[])
      n124 = And(x=w168, y=w172) -> (x .and. y?=w171:u16[])
      n125 = Divide(x=w171, y=256) -> (x/y=w167:dbl[])
      n126 = local read "Sampling rate"() -> (w149:i64)
      n127 = To Unsigned Byte Integer(number=w173) -> (unsigned 8bit integer=w170:u8[])
      n128 = To Unsigned Byte Integer(number=w167) -> (unsigned 8bit integer=w169:u8[])
      n129 = Build Array(w170, w169) -> (w166:u8[][])
      n130 = Number To Decimal String(number=w149) -> (decimal integer string=w147:string)  [unwired: 1 in]
      n131 = Transpose 2D Array(2D array=w166) -> (transposed array=w165:u8[][])
      n132 = Concatenate Strings(":FREQ:RAST ", w147) -> (w145:string)
      "concatenated string 2" <- w145
      n133 = Reshape Array(w165, w154) -> (w164:u8[])
      "output array" <- w164
      n134 = Type Cast(type="", x=w164) -> (*(type *) &x=w152:string)
      n135 = Build Array("INST 1\n:FUNC:MODE USER\n" ("write buffer"), w153, w152, w145, ":INIT:CONT OFF\n:TRIG:COUN 1\n:TRIG:DEL 0\n:TRIG:LEV 1.5\n:TRIG:MODE NORM\n:TRIG:SLOP POS\n:TRIG:SOUR:ADV EXT\n:TRIG:BURS ON\n:TRIG:STATE ON\n:VOLT:LEV:AMPL\\s1.2\n:OUTP ON" ("write buffer")) -> (w150:string[])
      "appended array" <- w150
      n136 = for {
        tunnel: _ -> [w189]
        tunnel: w150 -> [w188] mode=indexing
        shift-right: [w186] -> _
        shift-left: _ -> [w187]
        tunnel: [w185] -> _
        n137 = VISA Write(VISA resource name=w189, write buffer=w188, error in (no error)=w187) -> (VISA resource name out=w185:refnum<visa-resource-name>, error out=w186:errorcluster)  [unwired: 1 out]
        n138 = Wait (ms)(milliseconds to wait=u32 50) -> ()  [unwired: 1 out]
      }
    }
    frame Enabled {
    }
  }
  n139 = Format Value(string ("")="timing_v63-cwBlue_preset", format string="%02d", value (0)="Save as Preset #") -> (output string=w7:string)
  n140 = Concatenate Strings(w7, ".txt" ("string")) -> (w8:string)
  n141 = Concatenate Strings(w7, ".dat" ("string")) -> (w5:string)
  n142 = Build Path(base path=w4, name or relative path=w5) -> (appended path=→"appended path 2":path)
  n143 = Build Path(name or relative path=w8) -> ()  [unwired: 1 in, 1 out]
